vi "Main_MaintenanceCounters_V1.vi"() -> ()   [LabVIEW 2017]
panel:
  in  "LastCycleTimeCluster":cluster{"MachineName":string, "LastHour":string}
  out "LastCycleTimePath":path
  in  "CycleTimeArray":T1(array[cluster])
  in  "LastSeconds":i32
  out "ThisAppPath":path
  out "ModificationArray":string[](array[string])
  out "HourResetEnabled":string
  out "CycleCountHour":T2
  in  "ArrayCycleCountHour":T3(array[cluster])
  out "UserLevel":i32
  out "ServerConnectionStatus":string
  out "Line Name":string
  out "Array_BooleanMemoryPLC":T4(array[cluster])
  out "UserLogged":string
  in  "FormatCountersConfigArray":T5(array[cluster]) {"StoppageAlarmCounter" format="%#_6f"; "PreparationAlarmCounter" format="%#_6f"}
  out "CycleTimeCluster":T6
  out "Table Control":string[][](table)
  out "ConnectionCluster":cluster{"Connection":bool, "MachineName":string}
  out "UDT_1":T7
  in  "CountersConfiguration":T8
  out "CountersConfigMerged":T5(array[cluster])
  out "CounterLineName Path":path
  in  "Tab":T9(tab)
  in  "RefreshLists":bool
  in  "Selector_P#-Description":u16(ring) items=["104567 - Spinning Belt", "108724 - Emergency Stop", "105855 - Helicoil", "101415 - Inductive Sensor", "101111 - Magnetic Sensor"]
  in  "Selector_MachineSpareParts":u16(ring) items=["MA530", "MA520", "MA500-3", "MA500-2", "MA500-1", "MA490-2", "MA490-1", "MA475", "MA470", "MA455", "MA336", "MA335"]
  out "PathLocationMachineImage":path
  out "PathSparePartImage":path
  out "Image_LocationInMachine":T10(plugin-control)
  out "Image_SparePart":T10(plugin-control)
  in  "CountersConfigArray":T5(array[cluster]) {"StoppageAlarmCounter" format="%#_6f"; "PreparationAlarmCounter" format="%#_6f"}
  in  "RefreshCountersConfig":bool
  in  "SaveCountersConfig":bool
  out "Counters Configuration Path":path
  in  "MachineNameID":u16(ring) items=["MA530", "MA520", "MA500-3", "MA500-2", "MA500-1", "MA490-2", "MA490-1", "MA475", "MA470", "MA455", "MA336", "MA335"]
  in  "PLC Connection Array":T11(array[cluster]) {"PLC Type" items=["Keyence", "Allen Bradley", "Mitsubishi", "Panasonic", "Siemens"]}
  out "PLC Configuration Path":path
  in  "SavePLCConfig":bool
  in  "RefreshPLCConfig":bool
  in  "CreateTables":bool
  in  "EditUser":bool
  in  "GeneralParametersArray":cluster{"Parameter":string, "Value":string}[](array[cluster])
  in  "LoadDefaultConfig":bool
  in  "RemoveUser":bool
  in  "Logout":bool
  in  "Login":bool
  in  "AddUser":bool
  in  "GDrive":bool
  out "GeneralConfigPath":path
  in  "RefreshGeneralConfig":bool
  in  "SaveGeneralConfig":bool
  in  "ShowParetto":bool
  out "CycleTimeMonitor":T12(array[cluster])
  out "CycleTimePath":path
  out "legend":string[][](table)
  in  "Tab Control":T13(tab)
  in  "DictionaryArray":T14(array[cluster]) {"LifeCycle" format="%#_6f"}
  out "PathDictionary":path
  in  "SaveDictionary":bool
  in  "RefreshDictionary":bool
  in  "ResetAlarmButton":bool
  in  "QualityLogin":bool
  in  "MaintenanceLogin":bool
  in  "ResetAlarm":bool[](array[boolean])
  out "ArrayAlarm":bool[](array[boolean])
  out "OnlineStations":T15(array[cluster])
  in  "Counters Monitor Array":T16(array[cluster])
  out "CurrentCountersPath":path
  in  "Count Signal":bool[](array[boolean])
  in  "SaveCurrentCounter":bool
  in  "RefreshCurrentCounter":bool
  in  "Sort":bool
  out "Hour":string
  in  "stop":bool
  # "Cycles Based Maintenance"
  # "User"
  # "Line"
  # "Nidec Server Connection"
  # "Refresh Lists"
  # "Select Machine"
  # "Select PartNumber - Description"
  # "Location in the Machine"
  # "Spare Part Image"
  # "These paths are calculated automatically"
  # "Machine Name"
  # "Tool Crib P#"
  # "Description"
  # "SP1"
  # "SP2"
  # "Note:\nSP1 = Is the setpoint for the counter when the \nmachine will alert to prepare the replacement of\nthe component. This gives the technician time\nto get parts together.\n\nSP2 = Is the setpoint for the counter when the\nmachine will stop the operation until the part is \nreplaced, the operation can only be reset until\na quality employee comes to unlock with its \nuser and password."
  # "USER LEVEL 3 OR ABOVE TO ENABLE THIS CONFIGURATION IS NEEDED."
  # "Add the option to connect by serial port"
  # "Count Signal"
  # "Alarm Signal"
  # "Alarm Message"
  # "Machine Name"
  # "PLC Address"
  # "PLC Type"
  # "Value"
  # "Parameter"
  # "User Level 5 Requiered to View General Parameters"
  # "User Management"
  # "Idle Time: Is the maximum waiting time before a breakdown incidence is\nconsidered and created."
  # "Escalation Time: Is the maximum waiting time before sending an email \nto the escalation chain."
  # "Cycle Time Monitor"
  # "Cycle Time Monitor"
  # "Note: \nTo add a machine in this list of counters configuration it must be firt added in the PLC Connection tab."
  # "The SubAssembly can be either EOL, Motor, Stator, Rotor Etc, This is used to be able to crate several tables for the same line."
  # "buscar multiplos de ciclos para que coincidan \n\nestudiar investigacion de operaciones\n\nAgrupar las maquinas que trabajan en conjunto para agrupar tareas de mantenimiento.\nCambiar el metodo de seleccion de memorias de PLC usando solo strings para hacerlos universales."
  # "Nota para desarrollador: Revisar que al cerrar la incidencia se apague la alarma y se resetee el contador"
  # "1. Save counters to be loaded in the last state when the app starts up.\n\n2.Algorithm to read PLC counter values.\nthe key will be to set the signal from the PLC and reset from LabVIEW and the machine won't be able to start the new signal if the application has not been reset the previous one.\n\n3. Autosort getting the red status all the way up.\n\n4. Check cyle time between parts (The count signal must is the same for all the components in the same machine)"
  # "Component"
  # "Cycle Life"
  # "Manual"
  # "Un calculador de tiempo de vida en ciclos, que dependa del tipo de componente para calcular de acuerdo a la aplicacion.\n\npor ejemplo un slider, su tiempo de vida en es km de recorrido, midiendo cuanto se desplaza en cada movimiento, y cuantos desplazamientos hace por ciclo, se puede predecir, a los cuantos\nciclos va a fallar."
  # "Version:\nCBM V1.0\n03/03/2022 - 11:00\nEdgar Cruz\nMaintenance"
  # "MachineName"
  # "Tool Crib"
  # "ComponentName"
  # "Counter SetPoint"
  # "Actual"
  # "Status"
  # "Online Stations"
  # "Current Hour"
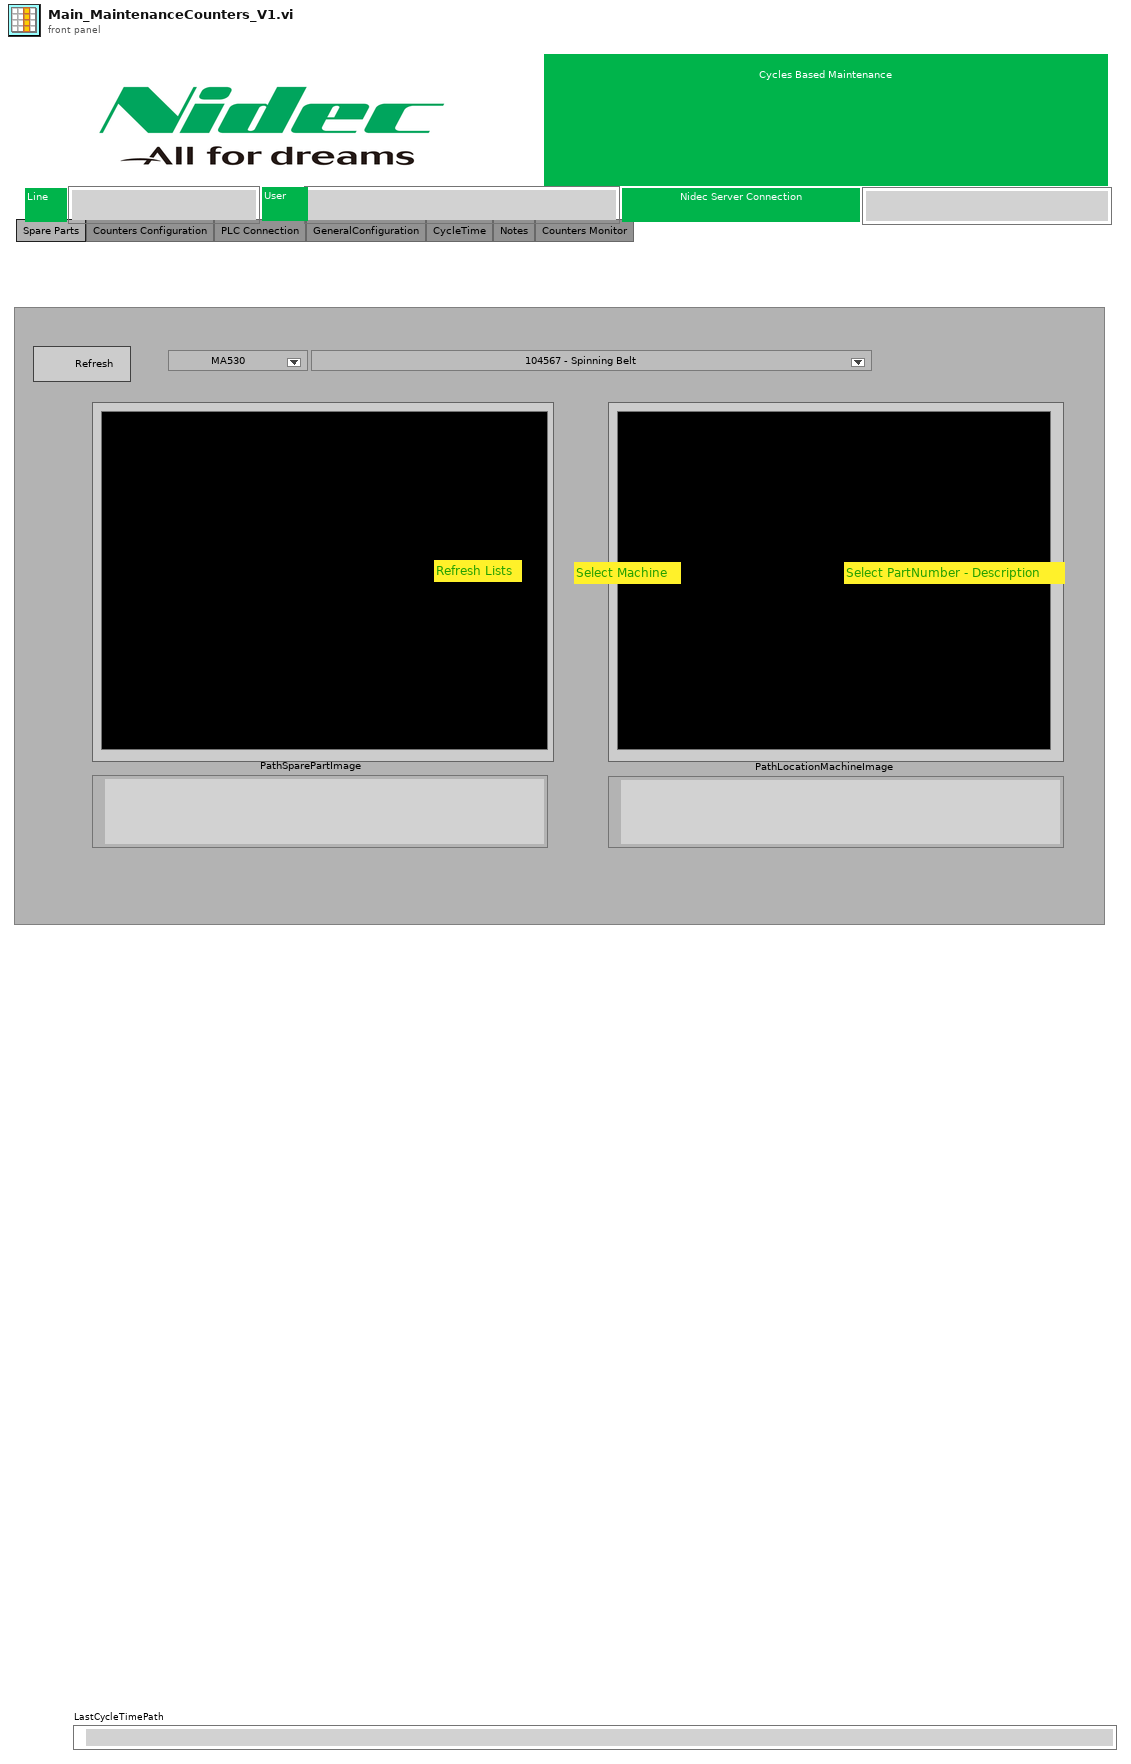
[diagram p1: front panel]
types:
  T1 = cluster{"MachineName":string, "LastHour":string}[]
  T2 = cluster{"MachineName":string, "HourLastCycle":string}
  T3 = cluster{"MachineName":string, "HourLastCycle":string}[]
  T4 = cluster{"PLC_Signal":bool, "MachineName":string}[]
  T5 = cluster{"ToolCribPartNumber":string, "ComponentName":string, "PreparationAlarmCounter":dbl, "StoppageAlarmCounter":dbl}[]
  T6 = cluster{"Connection":bool, "MachineName":string, "CycleTime":dbl}
  T7 = cluster{"ToolCribPartNumber":string, "ComponentName":string, "PreparationAlarmCounter":dbl, "StoppageAlarmCounter":dbl, "MachineName":string}
  T8 = cluster{"MachineName":string, "ComponentName":string, "StoppageAlarmCounter":dbl, "CurrentCount":dbl, "StatusColorBox":u32, "ToolCribPartNumber":string}
  T9 = enum32{"Spare Parts", "Counters Configuration", "PLC Connection", "GeneralConfiguration", "CycleTime", "Notes", "Counters Monitor"}
  T10 = typedef "IMAQ Image.ctl" = refnum<image>
  T11 = cluster{"MachineName":string, "PLC Address":string, "PLC Type":u16, "MemoryNumber1":string, "MemoryNumber2":string, "MemoryNumber3":string}[]
  T12 = cluster{"Connection":bool, "MachineName":string, "CycleTime":dbl}[]
  T13 = enum32{"Notes", "Dictionary", "Calculator", "Version Information"}
  T14 = cluster{"ComponentDescription":string, "LifeCycle":dbl, "ManualPDF":string}[]
  T15 = cluster{"Connection":bool, "MachineName":string}[]
  T16 = cluster{"MachineName":string, "ComponentName":string, "StoppageAlarmCounter":i32, "CurrentCount":i32, "StatusColorBox":u32, "ToolCribPartNumber":string}[]
  T17 = cluster{"ToolCribPartNumber":string, "ComponentName":string, "PreparationAlarmCounter":dbl, "StoppageAlarmCounter":dbl, "MachineName":string}[]
  T18 = cluster{"MachineName":string, "ComponentName":string, "StoppageAlarmCounter":i32, "CurrentCount":i32, "StatusColorBox":u32, "ToolCribPartNumber":string}
  T19 = enum8{"Enabled", "Disabled", "Disabled and Grayed Out"}
  T20 = typedef "Image Type" = u32
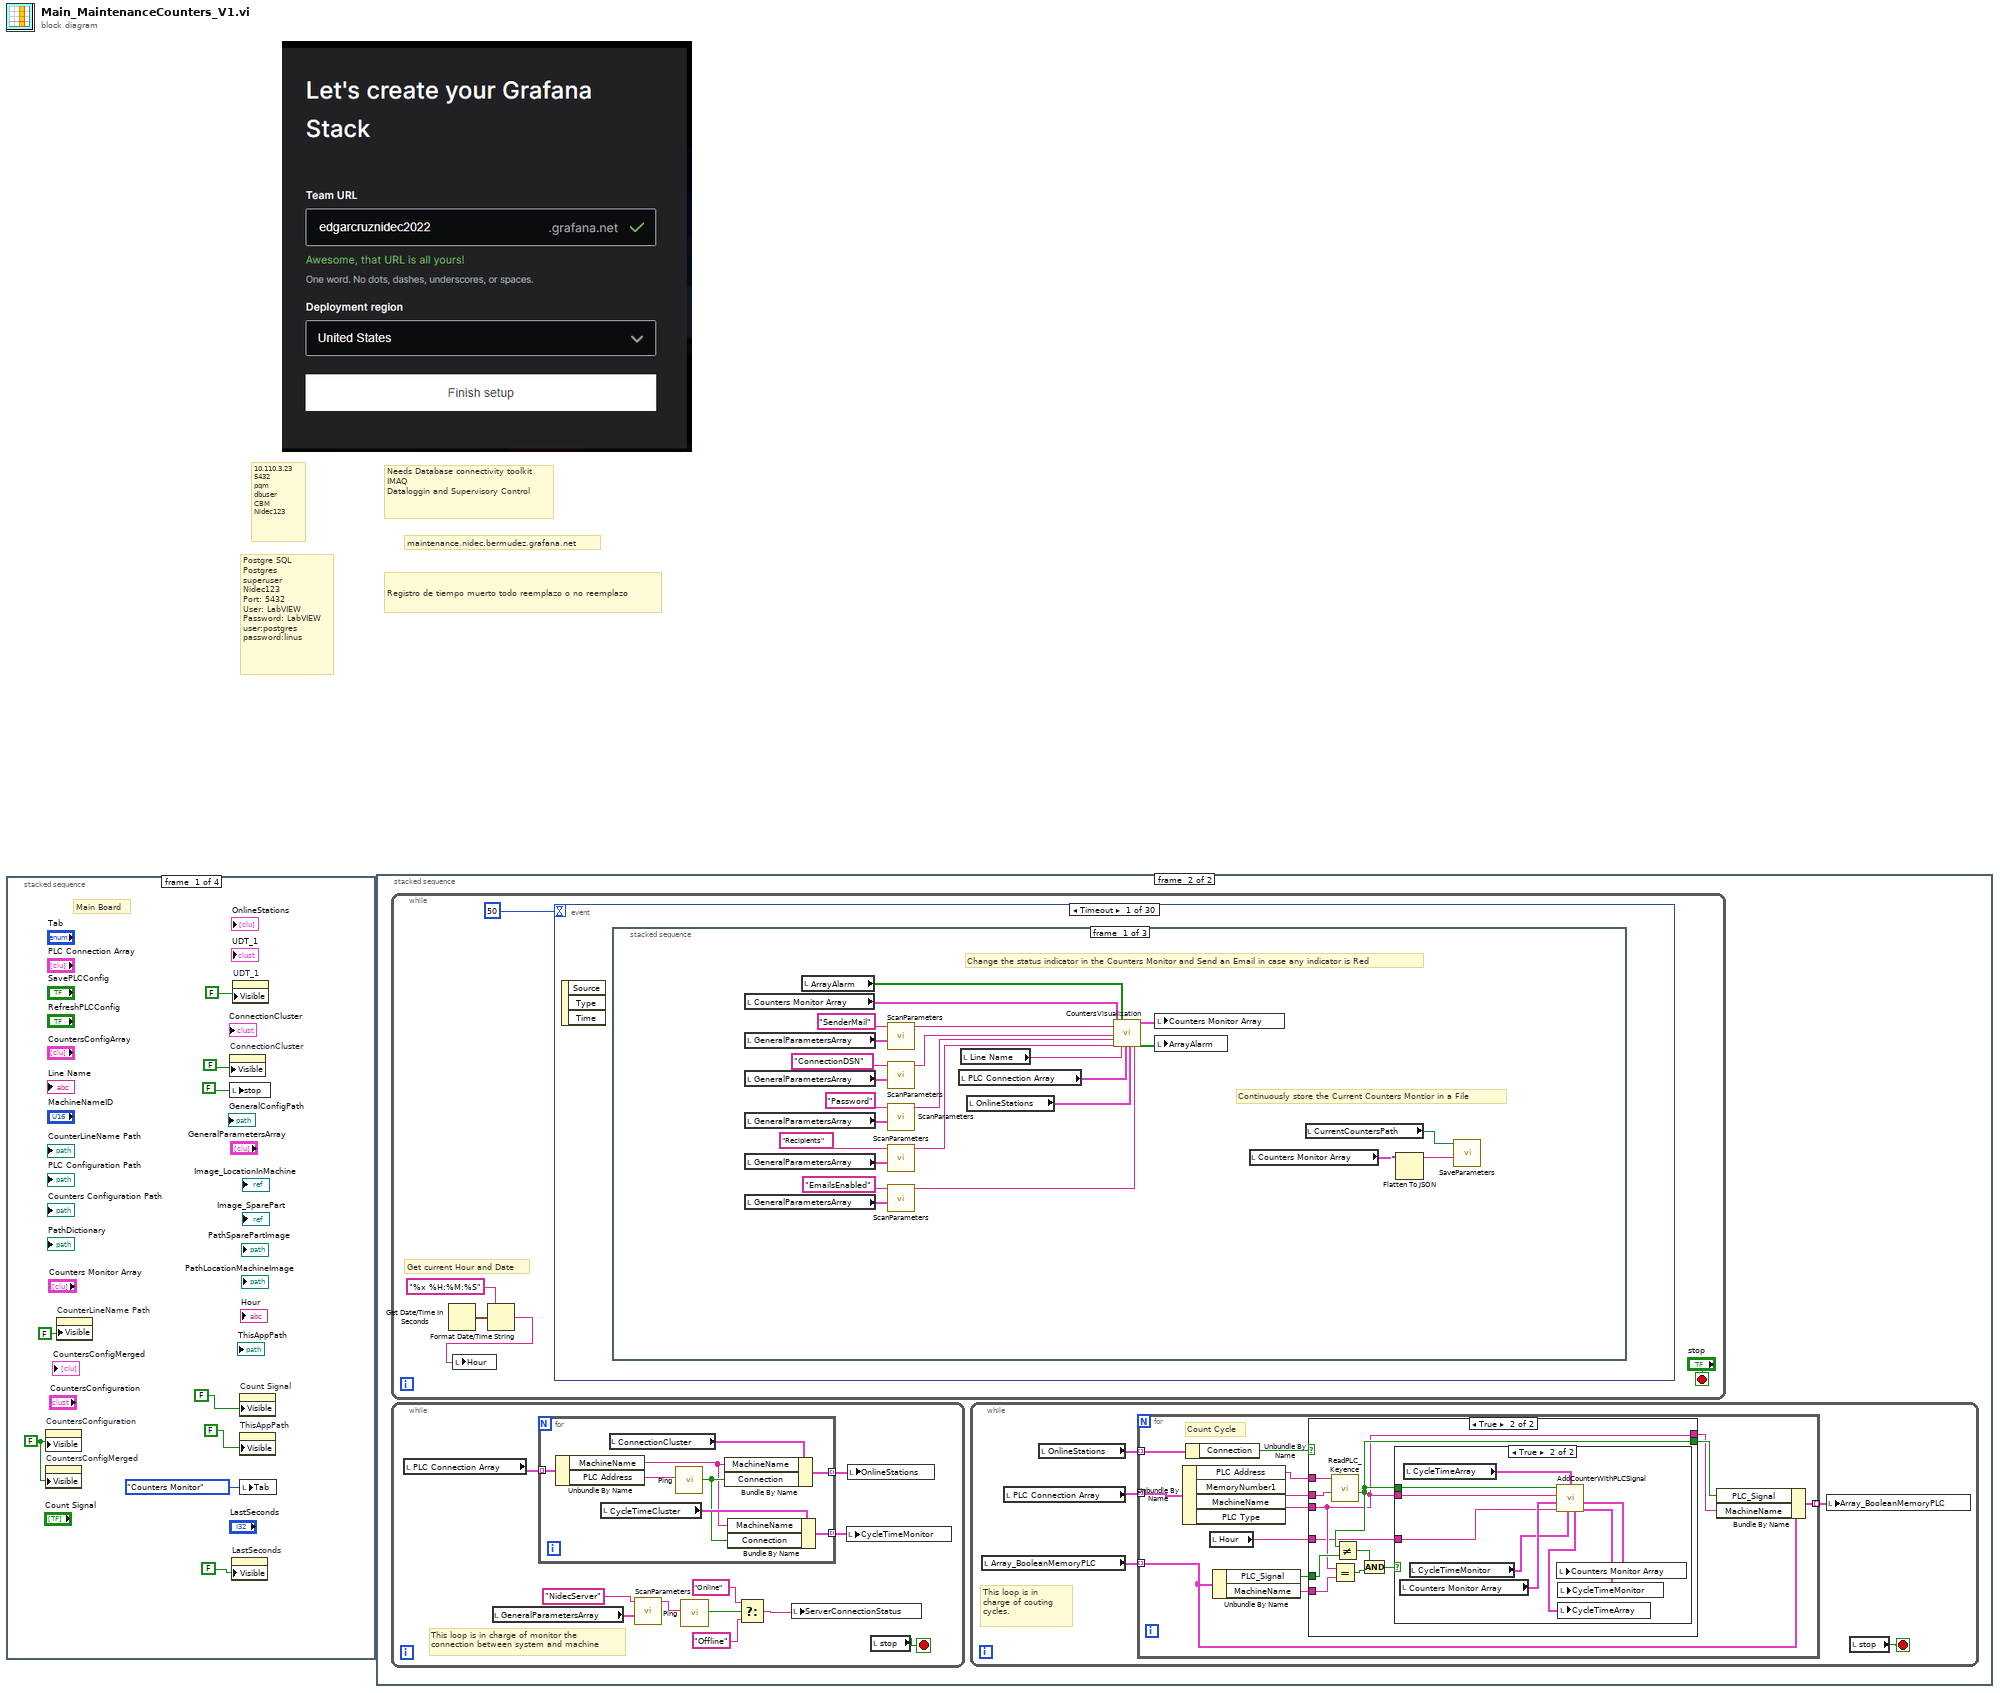
[diagram p0: block diagram]
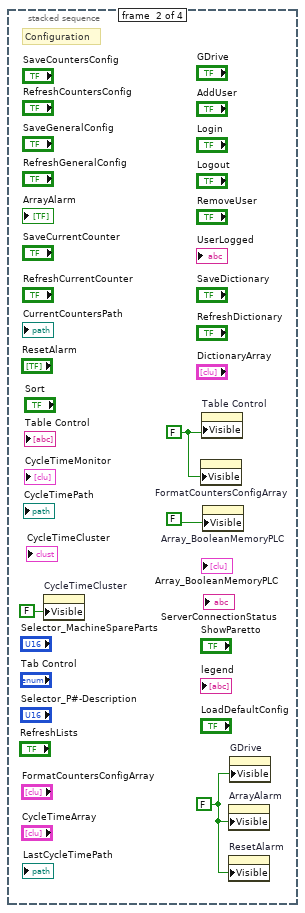
[diagram p2: hidden frame]
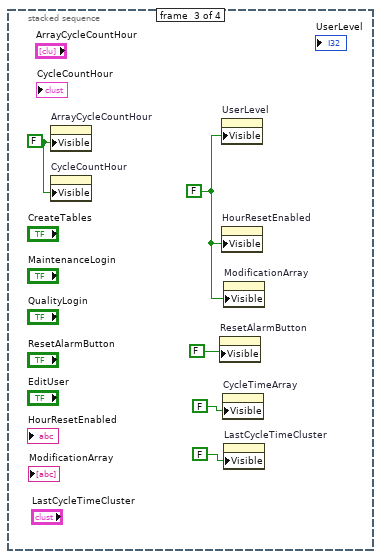
[diagram p3: hidden frame]
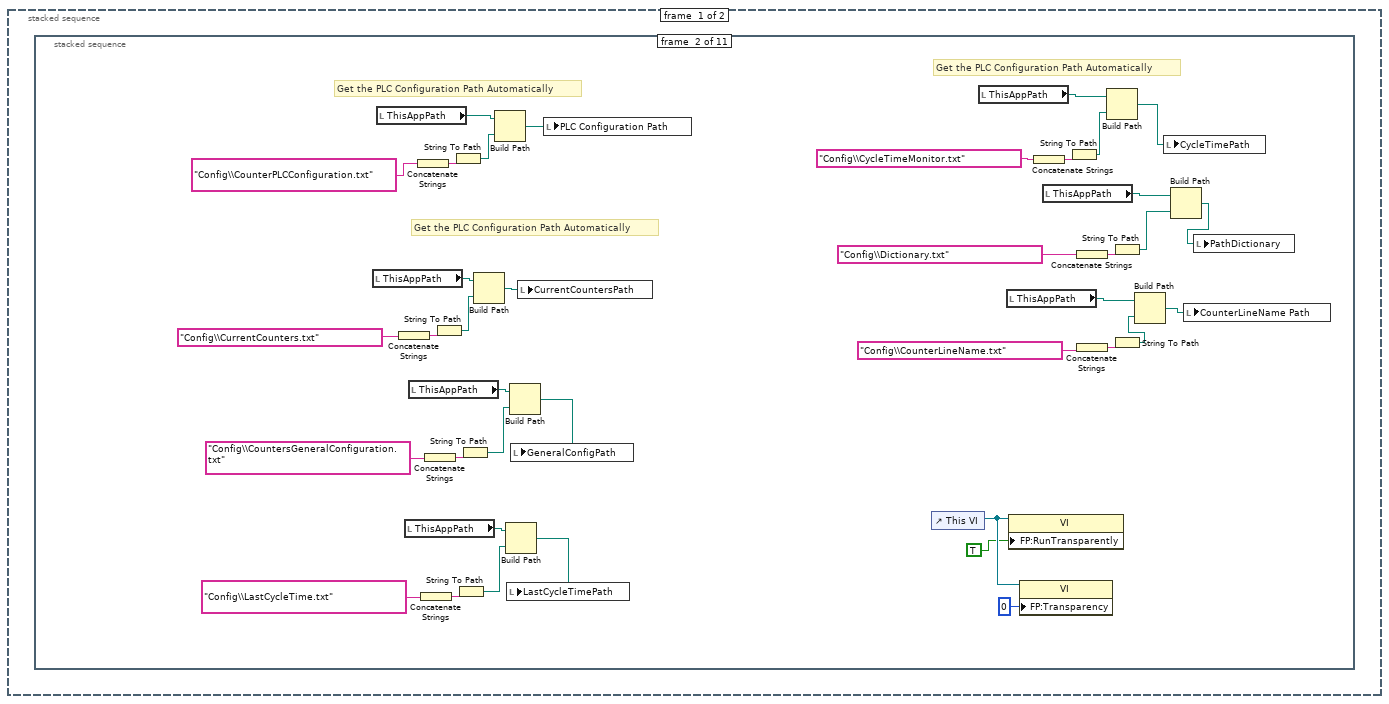
[diagram p5: hidden frame]
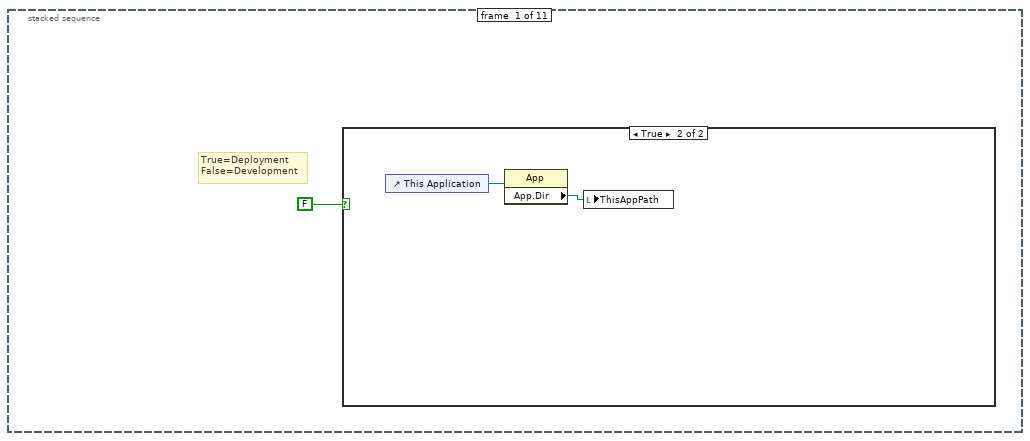
[diagram p6: hidden frame]
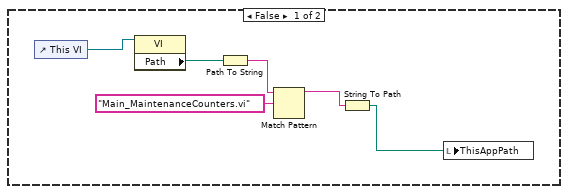
[diagram p7: hidden frame]
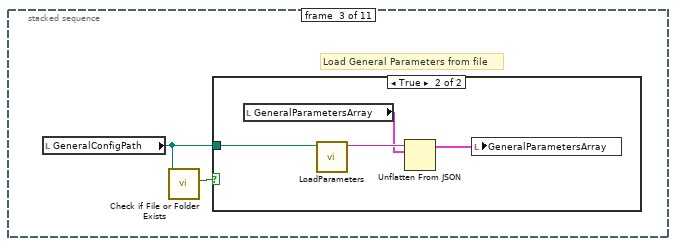
[diagram p8: hidden frame]
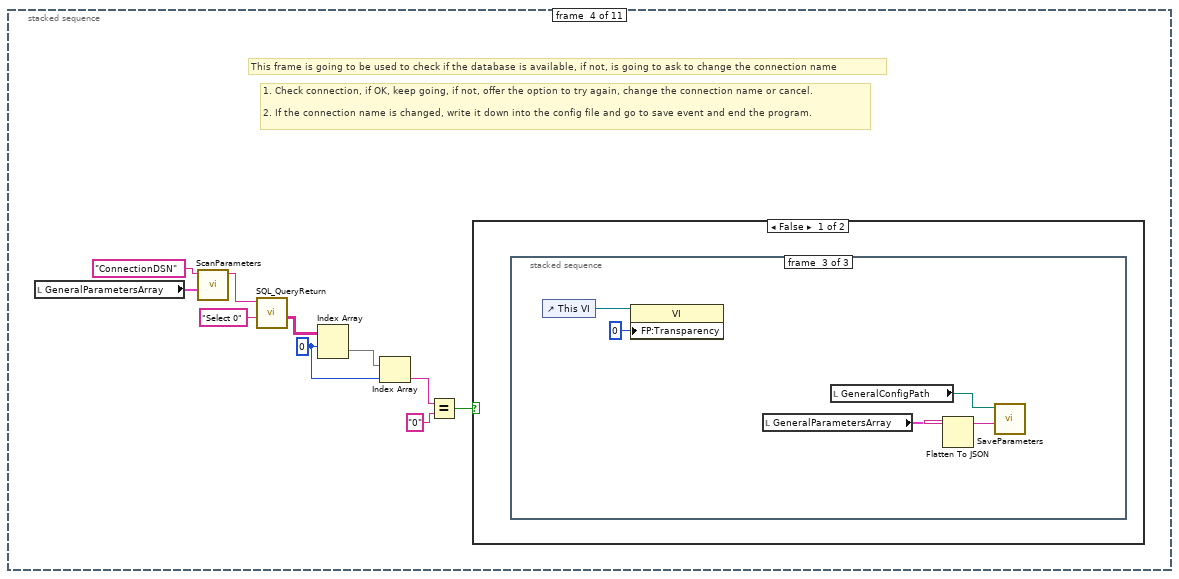
[diagram p10: hidden frame]
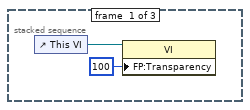
[diagram p11: hidden frame]
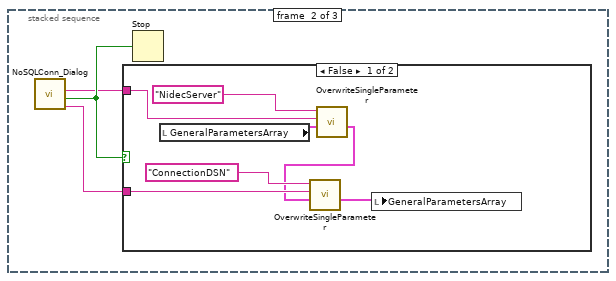
[diagram p12: hidden frame]
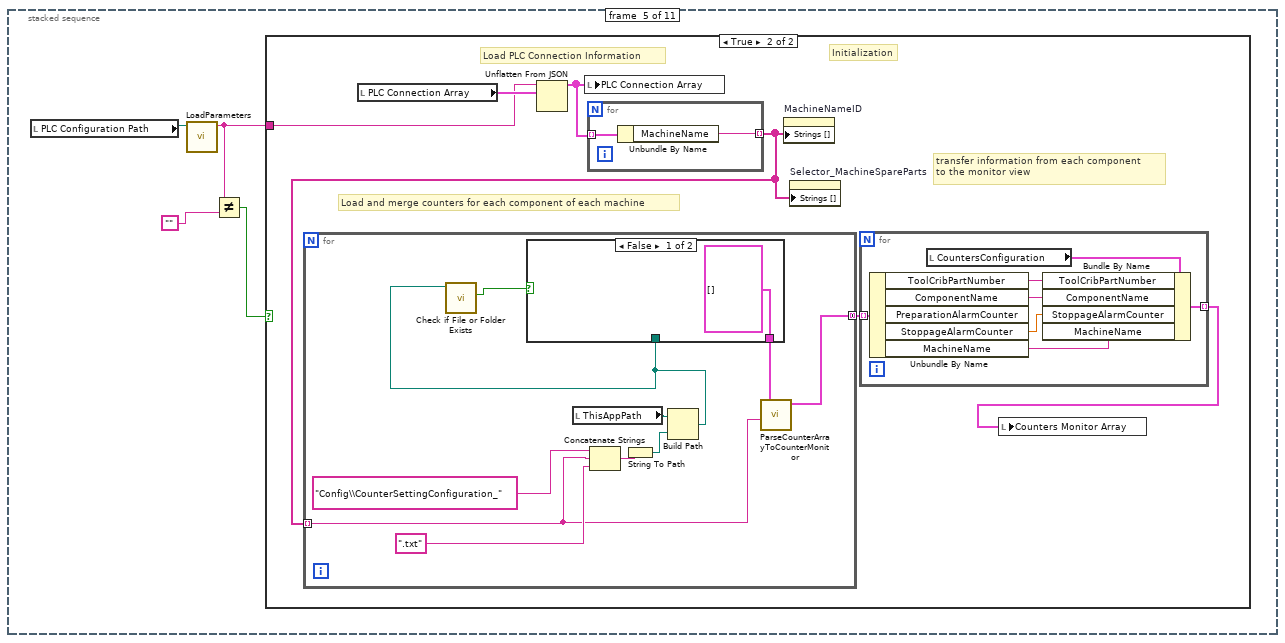
[diagram p15: hidden frame]
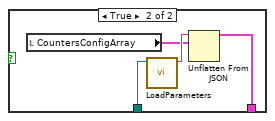
[diagram p17: hidden frame]
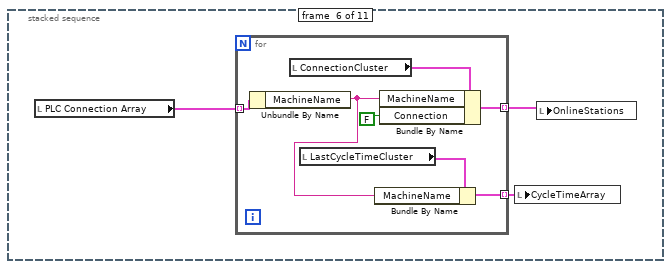
[diagram p18: hidden frame]
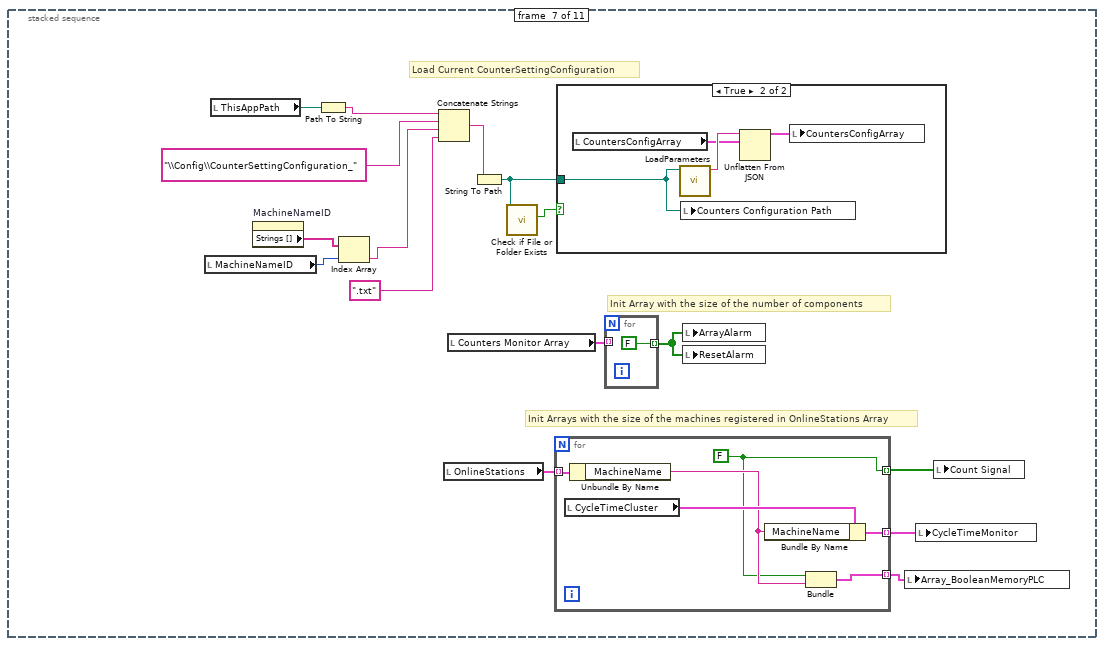
[diagram p19: hidden frame]
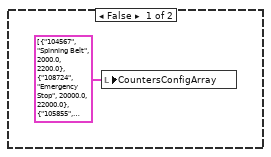
[diagram p20: hidden frame]
diagram:
  # "10.110.3.23\n5432\npqm\ndbuser\nCBM\nNidec123"
  # "maintenance.nidec.bermudez.grafana.net"
  # "Needs Database connectivity toolkit\nIMAQ\nDataloggin and Supervisory Control"
  # "Registro de tiempo muerto todo reemplazo o no reemplazo"
  # "Postgre SQL \nPostgres\nsuperuser\nNidec123\nPort: 5432\nUser: LabVIEW\nPassword: LabVIEW\nuser:postgres\npassword:linus"
  n1 = stacked-sequence {
    frame #0 {
      w8 = FALSE
      # "Main Board"
      n2 = property on="CountersConfiguration" class="Clust (strict)"("Visible"=w8) -> ()  [unwired: 2 in, 2 out]
      n3 = property on="CountersConfigMerged" class="Arr (strict)"("Visible"=w8) -> ()  [unwired: 2 in, 2 out]
      n4 = property on="CounterLineName Path" class="Path"("Visible"=FALSE) -> ()  [unwired: 2 in, 2 out]
      n5 = property on="ConnectionCluster" class="Clust (strict)"("Visible"=FALSE) -> ()  [unwired: 2 in, 2 out]
      n6 = local write "stop"(FALSE ("stop")) -> ()
      n7 = property on="LastSeconds" class="DigNum (strict)"("Visible"=FALSE) -> ()  [unwired: 2 in, 2 out]
      n8 = property on="UDT_1" class="Clust (strict)"("Visible"=FALSE) -> ()  [unwired: 2 in, 2 out]
      n9 = property on="Count Signal" class="Arr (strict)"("Visible"=FALSE) -> ()  [unwired: 2 in, 2 out]
      n10 = property on="ThisAppPath" class="Path"("Visible"=FALSE) -> ()  [unwired: 2 in, 2 out]
      n11 = local write "Tab"(T9."Counters Monitor" ("Tab")) -> ()
    }
    frame #1 {
      w11 = FALSE ("Visible")
      w12 = FALSE ("Visible")
      # "Configuration"
      n12 = property on="CycleTimeCluster" class="Clust (strict)"("Visible"=FALSE) -> ()  [unwired: 2 in, 2 out]
      n13 = property on="FormatCountersConfigArray" class="Arr (strict)"("Visible"=w12) -> ()  [unwired: 2 in, 2 out]
      n14 = property on="Table Control" class="Tbl (strict)"("Visible"=w12) -> ()  [unwired: 2 in, 2 out]
      n15 = property on="Array_BooleanMemoryPLC" class="Arr (strict)"("Visible"=FALSE) -> ()  [unwired: 2 in, 2 out]
      n16 = property on="ArrayAlarm" class="Arr (strict)"("Visible"=w11) -> ()  [unwired: 2 in, 2 out]
      n17 = property on="ResetAlarm" class="Arr (strict)"("Visible"=w11) -> ()  [unwired: 2 in, 2 out]
      n18 = property on="GDrive" class="Bool"("Visible"=w11) -> ()  [unwired: 2 in, 2 out]
    }
    frame #2 {
      w18 = FALSE
      w17 = FALSE
      n19 = property on="ArrayCycleCountHour" class="Arr (strict)"("Visible"=w18) -> ()  [unwired: 2 in, 2 out]
      n20 = property on="CycleCountHour" class="Clust (strict)"("Visible"=w18) -> ()  [unwired: 2 in, 2 out]
      n21 = property on="ResetAlarmButton" class="Bool"("Visible"=FALSE) -> ()  [unwired: 2 in, 2 out]
      n22 = property on="UserLevel" class="DigNum (strict)"("Visible"=w17) -> ()  [unwired: 2 in, 2 out]
      n23 = property on="HourResetEnabled" class="Str"("Visible"=w17) -> ()  [unwired: 2 in, 2 out]
      n24 = property on="CycleTimeArray" class="Arr (strict)"("Visible"=FALSE) -> ()  [unwired: 2 in, 2 out]
      n25 = property on="ModificationArray" class="Arr (strict)"("Visible"=w17) -> ()  [unwired: 2 in, 2 out]
      n26 = property on="LastCycleTimeCluster" class="Clust (strict)"("Visible"=FALSE) -> ()  [unwired: 2 in, 2 out]
    }
    frame #3 {
    }
  }
  n27 = stacked-sequence {
    frame #0 {
      n28 = stacked-sequence {
        frame #0 {
          # "True=Deployment\nFalse=Development"
          n29 = case shown="True" FALSE {
            frame False {
              n30 = control-ref of="This VI"() -> (w25:refnum<vi>)
              n31 = property class="VI"(reference=w25) -> ("Path"=w24:path)  [unwired: 1 in, 2 out]
              n32 = Path To String(path=w24) -> (string=w23:string)
              n33 = Match Pattern(string=w23, regular expression="Main_MaintenanceCounters.vi") -> (before substring=w21:string)  [unwired: 1 in, 3 out]
              n34 = String To Path(string=w21) -> (path=w20:path)
              n35 = local write "ThisAppPath"(w20) -> ()
            }
            frame True {
              n36 = control-ref of="This Application"() -> (w27:refnum<vi>)
              n37 = property class="App"(reference=w27) -> ("App.Dir"=w26:path)  [unwired: 1 in, 2 out]
              n38 = local write "ThisAppPath"(w26) -> ()
            }
          }
        }
        frame #1 {
          # "Get the PLC Configuration Path Automatically"
          # "Get the PLC Configuration Path Automatically"
          # "Get the PLC Configuration Path Automatically"
          n39 = local read "ThisAppPath"() -> (w47:path)
          n40 = local read "ThisAppPath"() -> (w49:path)
          n41 = Concatenate Strings("Config\\CurrentCounters.txt" ("regular expression")) -> (w62:string)
          n42 = local read "ThisAppPath"() -> (w30:path)
          n43 = local read "ThisAppPath"() -> (w44:path)
          n44 = Concatenate Strings("Config\\CounterPLCConfiguration.txt" ("regular expression")) -> (w65:string)
          n45 = Concatenate Strings("Config\\LastCycleTime.txt" ("regular expression")) -> (w28:string)
          n46 = Concatenate Strings("Config\\CountersGeneralConfiguration.txt" ("regular expression")) -> (w57:string)
          n47 = String To Path(string=w62) -> (path=w46:path)
          n48 = String To Path(string=w65) -> (path=w50:path)
          n49 = String To Path(string=w28) -> (path=w31:path)
          n50 = String To Path(string=w57) -> (path=w43:path)
          n51 = Build Path(base path=w47, name or relative path=w46) -> (appended path=w45:path)
          n52 = Build Path(base path=w49, name or relative path=w50) -> (appended path=w48:path)
          n53 = Build Path(base path=w30, name or relative path=w31) -> (appended path=w32:path)
          n54 = local write "LastCycleTimePath"(w32) -> ()
          n55 = Build Path(base path=w44, name or relative path=w43) -> (appended path=w42:path)
          n56 = local write "GeneralConfigPath"(w42) -> ()
          n57 = local write "CurrentCountersPath"(w45) -> ()
          n58 = local write "PLC Configuration Path"(w48) -> ()
          n59 = control-ref of="This VI"() -> (w53:refnum<vi>)
          n60 = local read "ThisAppPath"() -> (w41:path)
          n61 = local read "ThisAppPath"() -> (w35:path)
          n62 = property class="VI"(reference=w53, "FP:RunTransparently"=TRUE) -> ()  [unwired: 1 in, 2 out]
          n63 = property class="VI"(reference=w53, "FP:Transparency"=u8 0 ("Front Panel Window:Transparency")) -> ()  [unwired: 1 in, 2 out]
          n64 = Concatenate Strings("Config\\CycleTimeMonitor.txt" ("regular expression")) -> (w61:string)
          n65 = local read "ThisAppPath"() -> (w38:path)
          n66 = String To Path(string=w61) -> (path=w40:path)
          n67 = Concatenate Strings("Config\\Dictionary.txt" ("regular expression")) -> (w58:string)
          n68 = Concatenate Strings("Config\\CounterLineName.txt" ("regular expression")) -> (w55:string)
          n69 = Build Path(base path=w41, name or relative path=w40) -> (appended path=w39:path)
          n70 = String To Path(string=w58) -> (path=w37:path)
          n71 = String To Path(string=w55) -> (path=w34:path)
          n72 = Build Path(base path=w35, name or relative path=w34) -> (appended path=w33:path)
          n73 = local write "CycleTimePath"(w39) -> ()
          n74 = Build Path(base path=w38, name or relative path=w37) -> (appended path=w36:path)
          n75 = local write "CounterLineName Path"(w33) -> ()
          n76 = local write "PathDictionary"(w36) -> ()
        }
        frame #2 {
          # "Load General Parameters from file"
          n77 = local read "GeneralConfigPath"() -> (w66:path)
          n78 = call <vilib>:"Check if File or Folder Exists.vi"("path"=w66) -> ("file or folder exists?"=w67:bool)  [unwired: 8 in, 2 out]
          n79 = case shown="True" w67 {
            tunnel: w66 -> [_ w71]
            frame False {
            }
            frame True {
              n80 = local read "GeneralParametersArray"() -> (w69:cluster{"Parameter":string, "Value":string}[])
              n81 = call "LoadParameters.vi"("ShiftConfigPath"=w71) -> ("JSON_Text"=w70:string)  [unwired: 10 in]
              n82 = Unflatten From JSON(JSON string=w70, type and defaults=w69) -> (value=w68:cluster{"Parameter":string, "Value":string}[])  [unwired: 5 in, 1 out]
              n83 = local write "GeneralParametersArray"(w68) -> ()
            }
          }
        }
        frame #3 {
          w74 = 0 ("index (row)")
          # "1. Check connection, if OK, keep going, if not, offer the option to try again, change the connection name or cancel.\n\n2. If the connection name is changed, write it down into the config file and go to save event and end the program."
          # "This frame is going to be used to check if the database is available, if not, is going to ask to change the connection name"
          n84 = local read "GeneralParametersArray"() -> (w81:cluster{"Parameter":string, "Value":string}[])
          n85 = call "ScanParameters.vi"("MainConfigurationArray"=w81, "Parameter"="ConnectionDSN") -> ("Value"=w79:string)  [unwired: 9 in]
          n86 = call "SQL_QueryReturn.vi"("SQL query"="Select 0", "ConnectionDSN"=w79) -> ("data"=w77:string[][])  [unwired: 9 in]
          n87 = Index Array(array=w77, index (row)=w74) -> (element=w75:string[])  [unwired: 1 in]
          n88 = Index Array(array=w75, index=w74) -> (element=w73:string)
          n89 = Equal?(x=w73, y="0" ("SQL query")) -> (x = y?=w72:bool)
          n90 = case shown="False" w72 {
            frame False {
              n91 = stacked-sequence {
                frame #0 {
                  n92 = control-ref of="This VI"() -> (w82:refnum<vi>)
                  n93 = property class="VI"(reference=w82, "FP:Transparency"=u8 100 ("Front Panel Window:Transparency")) -> ()  [unwired: 1 in, 2 out]
                }
                frame #1 {
                  n94 = call "NoSQLConn_Dialog.vi"() -> ("NewDSN"=w86:string, "Boolean"=w85:bool, "NewIPAddress"=w84:string)  [unwired: 9 in]
                  n95 = case shown="False" w85 {
                    tunnel: w86 -> [w92 _]
                    tunnel: w84 -> [w89 _]
                    frame False {
                      n96 = local read "GeneralParametersArray"() -> (w90:cluster{"Parameter":string, "Value":string}[])
                      n97 = call "OverwriteSingleParameter.vi"("MainConfigurationArrayIN"=w90, "Value"=w89, "Parameter"="NidecServer") -> ("MainConfigurationArrayOUT"=w87:cluster{"Parameter":string, "Value":string}[])  [unwired: 8 in]
                      n98 = call "OverwriteSingleParameter.vi"("MainConfigurationArrayIN"=w87, "Value"=w92, "Parameter"="ConnectionDSN") -> ("MainConfigurationArrayOUT"=w88:cluster{"Parameter":string, "Value":string}[])  [unwired: 8 in]
                      n99 = local write "GeneralParametersArray"(w88) -> ()
                    }
                    frame True {
                    }
                  }
                  n100 = Stop(stop? (T)=w85) -> ()
                }
                frame #2 {
                  n101 = control-ref of="This VI"() -> (w98:refnum<vi>)
                  n102 = property class="VI"(reference=w98, "FP:Transparency"=u8 0 ("Front Panel Window:Transparency")) -> ()  [unwired: 1 in, 2 out]
                  n103 = local read "GeneralParametersArray"() -> (w94:cluster{"Parameter":string, "Value":string}[])
                  n104 = local read "GeneralConfigPath"() -> (w96:path)
                  n105 = Flatten To JSON(anything=w94) -> (JSON string=w95:string)  [unwired: 2 in, 1 out]
                  n106 = call "SaveParameters.vi"("JSON_Text"=w95, "ShiftConfigPath"=w96) -> ()  [unwired: 10 in]
                }
              }
            }
            frame True {
            }
          }
        }
        frame #4 {
          n107 = local read "PLC Configuration Path"() -> (w102:path)
          n108 = call "LoadParameters.vi"("ShiftConfigPath"=w102) -> ("JSON_Text"=w101:string)  [unwired: 10 in]
          n109 = Not Equal?(x=w101, y="") -> (x != y?=w99:bool)
          n110 = case shown="True" w99 {
            tunnel: w101 -> [_ w103]
            frame False {
            }
            frame True {
              # "Initialization"
              # "transfer information from each component\nto the monitor view"
              # "Load and merge counters for each component of each machine"
              # "Load PLC Connection Information"
              n111 = local read "PLC Connection Array"() -> (w108:T11)
              n112 = Unflatten From JSON(JSON string=w103, type and defaults=w108) -> (value=w107:T11)  [unwired: 5 in, 1 out]
              n113 = local write "PLC Connection Array"(w107) -> ()
              n114 = for {
                tunnel: w107 -> [w131] mode=indexing
                tunnel: [w132] -> w104 mode=indexing
                n115 = Unbundle By Name(w131) -> ("MachineName"=w132:string)
              }
              n116 = for {
                tunnel: w104 -> [w122] mode=indexing
                tunnel: [w121] -> w105 mode=concatenating
                n117 = local read "ThisAppPath"() -> (w118:path)
                n118 = Concatenate Strings("Config\\CounterSettingConfiguration_" ("regular expression"), w122, ".txt" ("regular expression")) -> (w125:string)
                n119 = String To Path(string=w125) -> (path=w117:path)
                n120 = Build Path(base path=w118, name or relative path=w117) -> (appended path=w116:path)
                n121 = call <vilib>:"Check if File or Folder Exists.vi"("path"=w116) -> ("file or folder exists?"=w120:bool)  [unwired: 8 in, 2 out]
                n122 = case shown="False" w120 {
                  tunnel: [T5 [] ("CountersConfigArray") w129] -> w119
                  tunnel: w116 -> [_ w128]
                  frame False {
                  }
                  frame True {
                    n123 = local read "CountersConfigArray"() -> (w127:T5)
                    n124 = call "LoadParameters.vi"("ShiftConfigPath"=w128) -> ("JSON_Text"=w130:string)  [unwired: 10 in]
                    n125 = Unflatten From JSON(JSON string=w130, type and defaults=w127) -> (value=w129:T5)  [unwired: 5 in, 1 out]
                  }
                }
                n126 = call "ParseCounterArrayToCounterMonitor.vi"("MachineID"=w122, "CountersConfigArray"=w119) -> ("CounterMonitorArray"=w121:T17)  [unwired: 9 in]
              }
              n127 = property on="MachineNameID" class="Ring (strict)"("Strings []"=w104) -> ()  [unwired: 2 in, 2 out]
              n128 = property on="Selector_MachineSpareParts" class="Ring (strict)"("Strings []"=w104) -> ()  [unwired: 2 in, 2 out]
              n129 = for {
                tunnel: [w113] -> w106 mode=indexing
                tunnel: w105 -> [w112] mode=indexing
                n130 = Unbundle By Name(w112) -> ("ToolCribPartNumber"=w111:string, "ComponentName"=w114:string, "StoppageAlarmCounter"=w110:dbl, "MachineName"=w109:string)  [unwired: 1 out]
                n131 = local read "CountersConfiguration"() -> (w115:T8)
                n132 = Bundle By Name(cluster=w115, "ToolCribPartNumber"=w111, "ComponentName"=w114, "StoppageAlarmCounter"=w110, "MachineName"=w109) -> (w113:T8)
              }
              n133 = local write "Counters Monitor Array"(w106) -> ()
            }
          }
        }
        frame #5 {
          n134 = local read "PLC Connection Array"() -> (w135:T11)
          n135 = for {
            tunnel: w135 -> [w142] mode=indexing
            tunnel: [w140] -> w134 mode=indexing
            tunnel: [w136] -> w133 mode=indexing
            n136 = Unbundle By Name(w142) -> ("MachineName"=w137:string)
            n137 = local read "ConnectionCluster"() -> (w141:cluster{"Connection":bool, "MachineName":string})
            n138 = local read "LastCycleTimeCluster"() -> (w138:cluster{"MachineName":string, "LastHour":string})
            n139 = Bundle By Name(cluster=w138, "MachineName"=w137) -> (w136:cluster{"MachineName":string, "LastHour":string})
            n140 = Bundle By Name(cluster=w141, "MachineName"=w137, "Connection"=FALSE) -> (w140:cluster{"Connection":bool, "MachineName":string})
          }
          n141 = local write "CycleTimeArray"(w133) -> ()
          n142 = local write "OnlineStations"(w134) -> ()
        }
        frame #6 {
          # "Load Current CounterSettingConfiguration"
          # "Init Array with the size of the number of components"
          # "Init Arrays with the size of the machines registered in OnlineStations Array"
          n143 = local read "MachineNameID"() -> (w158:u16)
          n144 = local read "ThisAppPath"() -> (w143:path)
          n145 = property on="MachineNameID" class="Ring (strict)"() -> ("Strings []"=w157:string[])  [unwired: 2 in, 2 out]
          n146 = Path To String(path=w143) -> (string=w144:string)
          n147 = Index Array(array=w157, index=w158) -> (element=w155:string)
          n148 = Concatenate Strings(w144, "\\Config\\CounterSettingConfiguration_" ("regular expression"), w155, ".txt" ("regular expression")) -> (w156:string)
          n149 = local read "OnlineStations"() -> (w148:T15)
          n150 = local read "Counters Monitor Array"() -> (w150:T16)
          n151 = String To Path(string=w156) -> (path=w153:path)
          n152 = call <vilib>:"Check if File or Folder Exists.vi"("path"=w153) -> ("file or folder exists?"=w154:bool)  [unwired: 8 in, 2 out]
          n153 = for {
            tunnel: w148 -> [w163] mode=indexing
            tunnel: [w160] -> w147 mode=indexing
            tunnel: [w162] -> w146 mode=indexing
            tunnel: [w159] -> w145 mode=indexing
            w160 = FALSE
            n154 = local read "CycleTimeCluster"() -> (w164:T6)
            n155 = Unbundle By Name(w163) -> ("MachineName"=w161:string)
            n156 = Bundle By Name(cluster=w164, "MachineName"=w161) -> (w162:T6)
            n157 = Bundle(w160, "MachineName"=w161) -> (w159:cluster{bool, "MachineName":string})  [unwired: 1 in]
          }
          n158 = case shown="True" w154 {
            tunnel: w153 -> [_ w169]
            frame False {
              n159 = local write "CountersConfigArray"(T5 [{"ToolCribPartNumber"="104567", "ComponentName"="Spinning Belt", "PreparationAlarmCounter"=2000.0, "StoppageAlarmCounter"=2200.0}, {"ToolCribPartNumber"="108724", "ComponentName"="Emergency Stop", "PreparationAlarmCounter"=20000.0, "StoppageAlarmCounter"=22000.0}, {"ToolCribPartNumber"="105855", "ComponentName"="Helicoil", "PreparationAlarmCounter"=38000.0, "StoppageAlarmCounter"=40000.0}, {"ToolCribPartNumber"="101415", "ComponentName"="NewPart", "PreparationAlarmCounter"=12000.0, "StoppageAlarmCounter"=12300.0}] ("CountersConfigArray")) -> ()
            }
            frame True {
              n160 = local read "CountersConfigArray"() -> (w168:T5)
              n161 = call "LoadParameters.vi"("ShiftConfigPath"=w169) -> ("JSON_Text"=w170:string)  [unwired: 10 in]
              n162 = local write "Counters Configuration Path"(w169) -> ()
              n163 = Unflatten From JSON(JSON string=w170, type and defaults=w168) -> (value=w167:T5)  [unwired: 5 in, 1 out]
              n164 = local write "CountersConfigArray"(w167) -> ()
            }
          }
          n165 = for {
            tunnel: w150 -> [_] mode=indexing
            tunnel: [FALSE] -> w149 mode=indexing
          }
          n166 = local write "ArrayAlarm"(w149) -> ()
          n167 = local write "ResetAlarm"(w149) -> ()
          n168 = local write "Array_BooleanMemoryPLC"(w145) -> ()
          n169 = local write "CycleTimeMonitor"(w146) -> ()
          n170 = local write "Count Signal"(w147) -> ()
        }
        frame #7 {
          # "Load Dictionary"
          n171 = local read "CurrentCountersPath"() -> (w177:path)
          n172 = local read "Counters Monitor Array"() -> (w175:T16)
          n173 = local read "PathDictionary"() -> (w171:path)
          n174 = call "LoadParameters.vi"("ShiftConfigPath"=w177) -> ("JSON_Text"=w176:string)  [unwired: 10 in]
          n175 = call <vilib>:"Check if File or Folder Exists.vi"("path"=w171) -> ("file or folder exists?"=w172:bool)  [unwired: 8 in, 2 out]
          n176 = Unflatten From JSON(JSON string=w176, type and defaults=w175) -> (value=w174:T16)  [unwired: 5 in, 1 out]
          n177 = for {
            tunnel: w175 -> [w183] mode=indexing
            tunnel: w174 -> [w184]
            tunnel: [w182] -> w173 mode=indexing
            n178 = Unbundle By Name(w183) -> ("MachineName"=w187:string, "ComponentName"=w186:string, "ToolCribPartNumber"=w185:string)
            n179 = for {
              tunnel: w187 -> [w200]
              tunnel: w186 -> [w199]
              tunnel: w185 -> [w198]
              tunnel: w184 -> [w201] mode=indexing
              shift-right: [w188] -> w182
              shift-left: w183 -> [w189]
              n180 = Unbundle By Name(w201) -> ("MachineName"=w190:string, "ComponentName"=w191:string, "ToolCribPartNumber"=w192:string, "CurrentCount"=w194:i32)
              n181 = Equal?(x=w200, y=w190) -> (x = y?=w196:bool)
              n182 = Equal?(x=w199, y=w191) -> (x = y?=w197:bool)
              n183 = Equal?(x=w198, y=w192) -> (x = y?=w195:bool)
              n184 = Compound Arithmetic op=AND(w196, w197, w195) -> (w193:bool)
              n185 = case shown="True" w193 {
                tunnel: w194 -> [_ w208]
                tunnel: w192 -> [_ w207]
                tunnel: w191 -> [_ w206]
                tunnel: w190 -> [_ w205]
                tunnel: w189 -> [w202 w204]
                tunnel: [w202 w203] -> w188
                frame False {
                }
                frame True {
                  n186 = Bundle By Name(cluster=w204, "MachineName"=w205, "ComponentName"=w206, "ToolCribPartNumber"=w207, "CurrentCount"=w208) -> (w203:T18)
                }
              }
            }
          }
          n187 = case shown="True" w172 {
            tunnel: w171 -> [_ w180]
            frame False {
            }
            frame True {
              n188 = local read "DictionaryArray"() -> (w181:T14)
              n189 = call "LoadParameters.vi"("ShiftConfigPath"=w180) -> ("JSON_Text"=w179:string)  [unwired: 10 in]
              n190 = Unflatten From JSON(JSON string=w179, type and defaults=w181) -> (value=w178:T14)  [unwired: 5 in, 1 out]
              n191 = local write "DictionaryArray"(w178) -> ()
            }
          }
          n192 = local write "Counters Monitor Array"(w173) -> ()
        }
        frame #8 {
          w213 = T19."Disabled and Grayed Out" ("Disabled")
          # "Logout and disable information"
          # "Load Line name from General parameters"
          n193 = local write "UserLevel"(0) -> ()
          n194 = local write "UserLogged"("") -> ()
          n195 = property on="PLC Connection Array" class="Arr (strict)"("DisabledEnum"=w213) -> ()  [unwired: 2 in, 2 out]
          n196 = property on="GeneralParametersArray" class="Arr (strict)"("Visible"=FALSE) -> ()  [unwired: 2 in, 2 out]
          n197 = property on="CountersConfigArray" class="Arr (strict)"("DisabledEnum"=w213) -> ()  [unwired: 2 in, 2 out]
          n198 = local read "GeneralParametersArray"() -> (w210:cluster{"Parameter":string, "Value":string}[])
          n199 = call "ScanParameters.vi"("MainConfigurationArray"=w210, "Parameter"="LineName") -> ("Value"=w211:string)  [unwired: 9 in]
          n200 = local write "Line Name"(w211) -> ()
        }
        frame #9 {
          # "This array must have one element per machine and register the hour \nso it must be initialized with the number of stations"
          n201 = local read "OnlineStations"() -> (w231:T15)
          n202 = for {
            tunnel: w231 -> [w235] mode=indexing
            tunnel: [w232] -> w230 mode=indexing
            n203 = Unbundle By Name(w235) -> ("MachineName"=w233:string)
            n204 = local read "CycleCountHour"() -> (w234:T2)
            n205 = Bundle By Name(cluster=w234, "MachineName"=w233) -> (w232:T2)
          }
          n206 = local read "GeneralParametersArray"() -> (w223:cluster{"Parameter":string, "Value":string}[])
          n207 = local read "GeneralParametersArray"() -> (w222:cluster{"Parameter":string, "Value":string}[])
          n208 = local write "ArrayCycleCountHour"(w230) -> ()
          n209 = local read "GeneralParametersArray"() -> (w228:cluster{"Parameter":string, "Value":string}[])
          n210 = call "ScanParameters.vi"("MainConfigurationArray"=w223, "Parameter"="LineName") -> ("Value"=w224:string)  [unwired: 9 in]
          n211 = call "ScanParameters.vi"("MainConfigurationArray"=w222, "Parameter"="SubAssembly") -> ("Value"=w225:string)  [unwired: 9 in]
          n212 = Concatenate Strings("update \"", w224, "_userlogged\" set \"useroperations\"='0',\"userquality\"='0' where \"subassembly\"='", w225, "'") -> (w226:string)
          n213 = call "ScanParameters.vi"("MainConfigurationArray"=w228, "Parameter"="ConnectionDSN") -> ("Value"=w229:string)  [unwired: 9 in]
          n214 = To Lower Case(string=w226) -> (all lower case string=w227:string)
          n215 = call "SQL_QueryNoReturn.vi"("SQL query"=w227, "ConnectionDSN"=w229) -> ()  [unwired: 10 in]
        }
        frame #10 {
          n216 = local read "GeneralParametersArray"() -> (w239:cluster{"Parameter":string, "Value":string}[])
          n217 = local read "GeneralParametersArray"() -> (w241:cluster{"Parameter":string, "Value":string}[])
          n218 = local read "GeneralParametersArray"() -> (w245:cluster{"Parameter":string, "Value":string}[])
          n219 = local read "Counters Monitor Array"() -> (w236:T16)
          n220 = call "ScanParameters.vi"("MainConfigurationArray"=w239, "Parameter"="SubAssembly") -> ("Value"=w237:string)  [unwired: 9 in]
          n221 = call "ScanParameters.vi"("MainConfigurationArray"=w241, "Parameter"="LineName") -> ("Value"=w240:string)  [unwired: 9 in]
          n222 = call "ScanParameters.vi"("MainConfigurationArray"=w245, "Parameter"="ConnectionDSN") -> ("Value"=w243:string)  [unwired: 9 in]
          n223 = call "SQL_StoreCountersMonitor.vi"("Counters Monitor Array"=w236, "SubAssembly"=w237, "LineName"=w240, "ConnectionDSN"=w243) -> ()  [unwired: 8 in]
        }
      }
    }
    frame #1 {
      n224 = while {
        stop <- "stop" stop-if-true
        # "Get current Hour and Date"
        n225 = Get Date/Time In Seconds() -> (seconds since 1Jan1904=w307:timestamp)
        n226 = Format Date/Time String(time format string (%c)="%x %H:%M:%S", seconds (now)=w307) -> (date/time string=w304:string)  [unwired: 1 in]
        n227 = local write "Hour"(w304) -> ()
        n228 = event shown="[0] Timeout" {
          selector: _ -> [_ _ _ _ _ _ _ _ _ _ _ _ _ _ _ _ _ _ _ _ _ _ _ _ _ _ _ _ _ _]
          dyn-events: _ -> [_ _ _ _ _ _ _ _ _ _ _ _ _ _ _ _ _ _ _ _ _ _ _ _ _ _ _ _ _ _]
          timeout: 50 -> [_ _ _ _ _ _ _ _ _ _ _ _ _ _ _ _ _ _ _ _ _ _ _ _ _ _ _ _ _ _]
          event Timeout {
            n229 = event-data() -> ()  [unwired: 1 in, 3 out]
            n230 = stacked-sequence {
              frame #0 {
                # "Continuously store the Current Counters Montior in a File"
                # "Change the status indicator in the Counters Monitor and Send an Email in case any indicator is Red"
                n231 = local read "Counters Monitor Array"() -> (w330:T16)
                n232 = local read "GeneralParametersArray"() -> (w321:cluster{"Parameter":string, "Value":string}[])
                n233 = local read "GeneralParametersArray"() -> (w312:cluster{"Parameter":string, "Value":string}[])
                n234 = local read "GeneralParametersArray"() -> (w320:cluster{"Parameter":string, "Value":string}[])
                n235 = local read "GeneralParametersArray"() -> (w317:cluster{"Parameter":string, "Value":string}[])
                n236 = local read "GeneralParametersArray"() -> (w325:cluster{"Parameter":string, "Value":string}[])
                n237 = local read "ArrayAlarm"() -> (w327:bool[])
                n238 = call "ScanParameters.vi"("MainConfigurationArray"=w321, "Parameter"="SenderMail") -> ("Value"=w316:string)  [unwired: 9 in]
                n239 = call "ScanParameters.vi"("MainConfigurationArray"=w312, "Parameter"="ConnectionDSN") -> ("Value"=w310:string)  [unwired: 9 in]
                n240 = call "ScanParameters.vi"("MainConfigurationArray"=w320, "Parameter"="Password") -> ("Value"=w315:string)  [unwired: 9 in]
                n241 = call "ScanParameters.vi"("MainConfigurationArray"=w317, "Parameter"="Recipients") -> ("Value"=w314:string)  [unwired: 9 in]
                n242 = call "ScanParameters.vi"("MainConfigurationArray"=w325, "Parameter"="EmailsEnabled") -> ("Value"=w323:string)  [unwired: 9 in]
                n243 = local read "PLC Connection Array"() -> (w309:T11)
                n244 = local read "Line Name"() -> (w328:string)
                n245 = local read "OnlineStations"() -> (w313:T15)
                n246 = call "CountersVisualization.vi"("Counters Monitor Array IN"=w330, "SenderMail"=w316, "ConnectionDSN"=w310, "Password"=w315, "Recipients"=w314, "ArrayAlarmIN"=w327, "LineName"=w328, "PLC Connection Array"=w309, "OnlineStations"=w313, "EmailsEnabled"=w323) -> ("Counters Monitor Array OUT"=w329:T16, "ArrayAlarmOUT"=w326:bool[])  [unwired: 8 in]
                n247 = local write "Counters Monitor Array"(w329) -> ()
                n248 = local write "ArrayAlarm"(w326) -> ()
                n249 = local read "Counters Monitor Array"() -> (w331:T16)
                n250 = local read "CurrentCountersPath"() -> (w333:path)
                n251 = Flatten To JSON(anything=w331) -> (JSON string=w332:string)  [unwired: 2 in, 1 out]
                n252 = call "SaveParameters.vi"("JSON_Text"=w332, "ShiftConfigPath"=w333) -> ()  [unwired: 10 in]
              }
              frame #1 {
                # "If the usser logged in is level 5, enables all the configurations"
                n253 = local read "UserLevel"() -> (w337:i32)
                n254 = Equal?(x=w337, y=5) -> (x = y?=w335:bool)
                n255 = property on="GeneralParametersArray" class="Arr (strict)"("Visible"=w335) -> ()  [unwired: 2 in, 2 out]
                n256 = property on="CreateTables" class="Bool"("Visible"=w335) -> ()  [unwired: 2 in, 2 out]
                n257 = property on="EditUser" class="Bool"("Visible"=w335) -> ()  [unwired: 2 in, 2 out]
                n258 = property on="LoadDefaultConfig" class="Bool"("Visible"=w335) -> ()  [unwired: 2 in, 2 out]
                n259 = property on="ResetAlarmButton" class="Bool"() -> ("Visible"=w334:bool)  [unwired: 2 in, 2 out]
                n260 = case shown="True" w334 {
                  frame False {
                  }
                  frame True {
                    n261 = stacked-sequence {
                      seq-local: [w346 _ _] -> [_ w362 _]
                      seq-local: [w342 _ _] -> [_ w361 _]
                      seq-local: [w339 _ _] -> [_ w360 _]
                      seq-local: [w345 _ _] -> [_ w359 _]
                      frame #0 {
                        n262 = local read "HourResetEnabled"() -> (w350:string)
                        n263 = local read "Hour"() -> (w358:string)
                        n264 = call <vilib>:"Space Constant.vi"() -> ("String"=w357:string)
                        n265 = call <vilib>:"Space Constant.vi"() -> ("String"=w351:string)
                        n266 = Match Pattern(string=w358, regular expression=w357) -> (after substring=w356:string)  [unwired: 1 in, 3 out]
                        n267 = Match Pattern(string=w350, regular expression=w351) -> (after substring=w352:string)  [unwired: 1 in, 3 out]
                        n268 = Match Pattern(string=w356, regular expression=":" ("time format string (%c)")) -> (before substring=w354:string, after substring=w344:string)  [unwired: 1 in, 2 out]
                        n269 = Match Pattern(string=w352, regular expression=":" ("time format string (%c)")) -> (before substring=w340:string, after substring=w338:string)  [unwired: 1 in, 2 out]
                        n270 = Match Pattern(string=w344, regular expression=":" ("time format string (%c)")) -> (before substring=w342:string)  [unwired: 1 in, 3 out]
                        n271 = Decimal String To Number(string=w354) -> (number=w349:i32)  [unwired: 2 in, 1 out]
                        n272 = Decimal String To Number(string=w340) -> (number=w348:i32)  [unwired: 2 in, 1 out]
                        n273 = Match Pattern(string=w338, regular expression=":" ("time format string (%c)")) -> (before substring=w339:string)  [unwired: 1 in, 3 out]
                        n274 = Subtract(x=w349, y=w348) -> (x-y=w345:i32)
                        n275 = Equal?(x=w345, y=0) -> (x = y?=w346:bool)
                      }
                      frame #1 {
                        # "Difference in hours"
                        # "Enabled minute"
                        # "Current minute"
                        n276 = case shown="True" w362 {
                          tunnel: w361 -> [w371 w389]
                          tunnel: w360 -> [w372 w388]
                          tunnel: w359 -> [w378 _]
                          frame False {
                            n277 = Match Pattern(string=w372, regular expression=":" ("time format string (%c)")) -> (before substring=w375:string)  [unwired: 1 in, 3 out]
                            n278 = Match Pattern(string=w371, regular expression=":" ("time format string (%c)")) -> (before substring=w376:string)  [unwired: 1 in, 3 out]
                            n279 = Multiply(x=w378, y=60) -> (x*y=w369:i32)
                            n280 = Decimal String To Number(string=w375) -> (number=w370:i32)  [unwired: 2 in, 1 out]
                            n281 = Decimal String To Number(string=w376) -> (number=w368:i32)  [unwired: 2 in, 1 out]
                            n282 = Subtract(x=w369, y=w370) -> (x-y=w367:i32)
                            n283 = Add(x=w367, y=w368) -> (x+y=w366:i32)
                            n284 = Greater Or Equal?(x=5 ("y"), y=w366) -> (x >= y?=w364:bool)
                            n285 = Not(x=w364) -> (.not. x?=w363:bool)
                            n286 = property on="ResetAlarmButton" class="Bool"("Visible"=w363) -> ()  [unwired: 2 in, 2 out]
                          }
                          frame True {
                            n287 = Match Pattern(string=w389, regular expression=":" ("time format string (%c)")) -> (before substring=w386:string)  [unwired: 1 in, 3 out]
                            n288 = Match Pattern(string=w388, regular expression=":" ("time format string (%c)")) -> (before substring=w385:string)  [unwired: 1 in, 3 out]
                            n289 = Decimal String To Number(string=w386) -> (number=w384:i32)  [unwired: 2 in, 1 out]
                            n290 = Decimal String To Number(string=w385) -> (number=w383:i32)  [unwired: 2 in, 1 out]
                            n291 = Subtract(x=w384, y=w383) -> (x-y=w381:i32)
                            n292 = Greater Or Equal?(x=w381, y=5) -> (x >= y?=w380:bool)
                            n293 = Not(x=w380) -> (.not. x?=w379:bool)
                            n294 = property on="ResetAlarmButton" class="Bool"("Visible"=w379) -> ()  [unwired: 2 in, 2 out]
                          }
                        }
                      }
                      frame #2 {
                        n295 = property on="ResetAlarmButton" class="Bool"() -> ("Visible"=w391:bool)  [unwired: 2 in, 2 out]
                        n296 = case shown="False" w391 {
                          frame False {
                            n297 = local read "GeneralParametersArray"() -> (w399:cluster{"Parameter":string, "Value":string}[])
                            n298 = local read "GeneralParametersArray"() -> (w398:cluster{"Parameter":string, "Value":string}[])
                            n299 = local read "GeneralParametersArray"() -> (w404:cluster{"Parameter":string, "Value":string}[])
                            n300 = call "ScanParameters.vi"("MainConfigurationArray"=w399, "Parameter"="LineName") -> ("Value"=w400:string)  [unwired: 9 in]
                            n301 = call "ScanParameters.vi"("MainConfigurationArray"=w398, "Parameter"="SubAssembly") -> ("Value"=w401:string)  [unwired: 9 in]
                            n302 = Concatenate Strings("update \"", w400, "_userlogged\" set \"useroperations\"='0',\"userquality\"='0' where \"subassembly\"='", w401, "'") -> (w402:string)
                            n303 = call "ScanParameters.vi"("MainConfigurationArray"=w404, "Parameter"="ConnectionDSN") -> ("Value"=w405:string)  [unwired: 9 in]
                            n304 = To Lower Case(string=w402) -> (all lower case string=w403:string)
                            n305 = call "SQL_QueryNoReturn.vi"("SQL query"=w403, "ConnectionDSN"=w405) -> ()  [unwired: 10 in]
                          }
                          frame True {
                          }
                        }
                      }
                    }
                  }
                }
              }
              frame #2 {
                w410 = ":" ("regular expression")
                # "Updates de SQL Table with the current values of the counters monitor each minute"
                n306 = local read "Hour"() -> (w412:string)
                n307 = Match Pattern(string=w412, regular expression=w410) -> (after substring=w411:string)  [unwired: 1 in, 3 out]
                n308 = Match Pattern(string=w411, regular expression=w410) -> (after substring=w409:string)  [unwired: 1 in, 3 out]
                n309 = Decimal String To Number(string=w409) -> (number=w408:i32)  [unwired: 2 in, 1 out]
                n310 = Equal?(x=w408, y=1) -> (x = y?=w407:bool)
                n311 = case shown="True" w407 {
                  frame False {
                  }
                  frame True {
                    n312 = stacked-sequence {
                      frame #0 {
                        n313 = local read "GeneralParametersArray"() -> (w422:cluster{"Parameter":string, "Value":string}[])
                        n314 = local read "GeneralParametersArray"() -> (w416:cluster{"Parameter":string, "Value":string}[])
                        n315 = local read "GeneralParametersArray"() -> (w418:cluster{"Parameter":string, "Value":string}[])
                        n316 = local read "Counters Monitor Array"() -> (w413:T16)
                        n317 = call "ScanParameters.vi"("MainConfigurationArray"=w422, "Parameter"="ConnectionDSN") -> ("Value"=w420:string)  [unwired: 9 in]
                        n318 = call "ScanParameters.vi"("MainConfigurationArray"=w416, "Parameter"="SubAssembly") -> ("Value"=w414:string)  [unwired: 9 in]
                        n319 = call "ScanParameters.vi"("MainConfigurationArray"=w418, "Parameter"="LineName") -> ("Value"=w417:string)  [unwired: 9 in]
                        n320 = call "SQL_CountersMonitorUpdate.vi"("Counters Monitor Array"=w413, "SubAssembly"=w414, "LineName"=w417, "ConnectionDSN"=w420) -> ()  [unwired: 8 in]
                      }
                      frame #1 {
                        n321 = local read "CycleTimeArray"() -> (w425:T1)
                        n322 = local read "LastCycleTimePath"() -> (w423:path)
                        n323 = Flatten To JSON(anything=w425) -> (JSON string=w424:string)  [unwired: 2 in, 1 out]
                        n324 = call "SaveParameters.vi"("JSON_Text"=w424, "ShiftConfigPath"=w423) -> ()  [unwired: 10 in]
                      }
                    }
                  }
                }
              }
            }
          }
          event "SavePLCConfig": Value Change {
            n325 = event-data() -> ()  [unwired: 1 in, 6 out]
            n326 = stacked-sequence {
              frame #0 {
                # "Checks if any parameter was changed and stores the changes in the Modification Array to Store modifications in database"
                n327 = local read "PLC Configuration Path"() -> (w434:path)
                n328 = local read "PLC Connection Array"() -> (w431:T11)
                n329 = local read "UserLogged"() -> (w430:string)
                n330 = call "LoadParameters.vi"("ShiftConfigPath"=w434) -> ("JSON_Text"=w433:string)  [unwired: 10 in]
                n331 = Unflatten From JSON(JSON string=w433, type and defaults=w431) -> (value=w432:T11)  [unwired: 5 in, 1 out]
                n332 = Match Pattern(string=w430, regular expression=",") -> (before substring=w428:string)  [unwired: 1 in, 3 out]
                n333 = for {
                  tunnel: w432 -> [w457] mode=indexing
                  tunnel: w431 -> [w456] mode=indexing
                  tunnel: w428 -> [w439]
                  shift-right: [w435] -> w426
                  shift-left: string[] [] -> [w436]
                  # "Before"
                  n334 = Unbundle By Name(w457) -> ("MachineName"=w454:string, "PLC Address"=w453:string, "PLC Type"=w455:u16, "MemoryNumber1"=w451:string, "MemoryNumber2"=w450:string, "MemoryNumber3"=w449:string)
                  n335 = Unbundle By Name(w456) -> ("MachineName"=w448:string, "PLC Address"=w447:string, "PLC Type"=w446:u16, "MemoryNumber1"=w444:string, "MemoryNumber2"=w443:string, "MemoryNumber3"=w442:string)
                  n336 = Number To Decimal String(number=w455) -> (decimal integer string=w452:string)  [unwired: 1 in]
                  n337 = Number To Decimal String(number=w446) -> (decimal integer string=w445:string)  [unwired: 1 in]
                  n338 = Build Array(w454, w453, w452, w451, w450, w449) -> (w438:string[])
                  n339 = Build Array(w448, w447, w445, w444, w443, w442) -> (w437:string[])
                  n340 = Not Equal?(x=w438, y=w437) -> (x != y?=w441:bool[])
                  n341 = Or Array Elements(Boolean array=w441) -> (logical OR=w440:bool)
                  n342 = case shown="True" w440 {
                    tunnel: w439 -> [_ w460]
                    tunnel: w438 -> [_ w462]
                    tunnel: w437 -> [_ w461]
                    tunnel: [w458 w459] -> w435
                    tunnel: w436 -> [w458 w463]
                    frame False {
                    }
                    frame True {
                      n343 = call "SQL_SortModifications.vi"("UserLogged"=w460, "AfterArray"=w461, "BeforeArray"=w462, "CleanArray"=w463) -> ("ResultArray"=w459:string[])  [unwired: 7 in]
                    }
                  }
                }
                n344 = local write "ModificationArray"(w426) -> ()
              }
              frame #1 {
                n345 = Get Date/Time In Seconds() -> (seconds since 1Jan1904=w468:timestamp)
                n346 = local read "UserLogged"() -> (w471:string)
                n347 = local read "ModificationArray"() -> (w472:string[])
                n348 = Format Date/Time String(time format string (%c)="%x", seconds (now)=w468) -> (date/time string=w466:string)  [unwired: 1 in]
                n349 = Format Date/Time String(time format string (%c)="%H:%M:%S", seconds (now)=w468) -> (date/time string=w465:string)  [unwired: 1 in]
                n350 = Match Pattern(string=w471, regular expression=",") -> (before substring=w464:string)  [unwired: 1 in, 3 out]
                n351 = for {
                  tunnel: w472 -> [w476] mode=indexing
                  tunnel: w466 -> [w480]
                  tunnel: w465 -> [w479]
                  tunnel: w464 -> [w478]
                  w477 = "','"
                  n352 = local read "GeneralParametersArray"() -> (w484:cluster{"Parameter":string, "Value":string}[])
                  n353 = local read "GeneralParametersArray"() -> (w488:cluster{"Parameter":string, "Value":string}[])
                  n354 = call "ScanParameters.vi"("MainConfigurationArray"=w484, "Parameter"="LineName") -> ("Value"=w482:string)  [unwired: 9 in]
                  n355 = call "ScanParameters.vi"("MainConfigurationArray"=w488, "Parameter"="ConnectionDSN") -> ("Value"=w486:string)  [unwired: 9 in]
                  n356 = Concatenate Strings("insert into \"", w482, "_systemlog\" values('", w480, w477, w479, w477, w478, w477, w476, "')") -> (w474:string)
                  n357 = To Lower Case(string=w474) -> (all lower case string=w473:string)
                  n358 = call "SQL_QueryNoReturn.vi"("SQL query"=w473, "ConnectionDSN"=w486) -> ()  [unwired: 10 in]
                }
              }
              frame #2 {
                # "Store the PLC Configuration in JSON File"
                n359 = local read "PLC Connection Array"() -> (w500:T11)
                n360 = local read "PLC Configuration Path"() -> (w499:path)
                n361 = Flatten To JSON(anything=w500) -> (JSON string=w498:string)  [unwired: 2 in, 1 out]
                n362 = local read "GeneralParametersArray"() -> (w494:cluster{"Parameter":string, "Value":string}[])
                n363 = local read "GeneralParametersArray"() -> (w490:cluster{"Parameter":string, "Value":string}[])
                n364 = call "SaveParameters.vi"("JSON_Text"=w498, "ShiftConfigPath"=w499) -> ()  [unwired: 10 in]
                n365 = call "ScanParameters.vi"("MainConfigurationArray"=w494, "Parameter"="ConnectionDSN") -> ("Value"=w492:string)  [unwired: 9 in]
                n366 = call "ScanParameters.vi"("MainConfigurationArray"=w490, "Parameter"="LineName") -> ("Value"=w489:string)  [unwired: 9 in]
                n367 = for {
                  tunnel: w500 -> [w504] mode=indexing
                  tunnel: [w501] -> w495 mode=indexing
                  tunnel: w492 -> [w503]
                  tunnel: w489 -> [w502]
                  n368 = Unbundle By Name(w504) -> ("MachineName"=w501:string)
                  n369 = disable-structure shown="Disabled" {
                    disable-tunnel: w503 -> [w508 _]
                    disable-tunnel: w502 -> [w506 _]
                    disable-tunnel: w501 -> [w505 _]
                    frame Disabled {
                      n370 = call "SQL_CycleTime_RegisterMachine.vi"("MachineName"=w505, "LineName"=w506, "TableName"="CycleTime", "ConnectionDSN"=w508) -> ()  [unwired: 8 in]
                    }
                    frame Enabled {
                    }
                  }
                }
                n371 = local read "CounterLineName Path"() -> (w496:path)
                n372 = local read "Line Name"() -> (w497:string)
                n373 = call "SaveParameters.vi"("JSON_Text"=w497, "ShiftConfigPath"=w496) -> ()  [unwired: 10 in]
                n374 = property on="MachineNameID" class="Ring (strict)"("Strings []"=w495) -> ()  [unwired: 2 in, 2 out]
                n375 = property on="Selector_MachineSpareParts" class="Ring (strict)"("Strings []"=w495) -> ()  [unwired: 2 in, 2 out]
              }
            }
          }
          event "SaveCountersConfig": Value Change {
            n376 = event-data() -> ()  [unwired: 1 in, 6 out]
            n377 = stacked-sequence {
              frame #0 {
                n378 = local read "ThisAppPath"() -> (w510:path)
                n379 = local read "MachineNameID"() -> (w517:u16)
                n380 = property on="MachineNameID" class="Ring (strict)"() -> ("Strings []"=w516:string[])  [unwired: 2 in, 2 out]
                n381 = Path To String(path=w510) -> (string=w509:string)
                n382 = Index Array(array=w516, index=w517) -> (element=w514:string)
                n383 = Concatenate Strings(w509, "\\Config\\CounterSettingConfiguration_" ("regular expression"), w514, ".txt" ("regular expression")) -> (w515:string)
                n384 = String To Path(string=w515) -> (path=w513:path)
                n385 = local write "Counters Configuration Path"(w513) -> ()
              }
              frame #1 {
                # "Checks if any parameter was changed and stores the changes in the Modification Array to Store modifications in database"
                n386 = local read "Counters Configuration Path"() -> (w526:path)
                n387 = local read "CountersConfigArray"() -> (w523:T5)
                n388 = local read "UserLogged"() -> (w522:string)
                n389 = call "LoadParameters.vi"("ShiftConfigPath"=w526) -> ("JSON_Text"=w525:string)  [unwired: 10 in]
                n390 = Unflatten From JSON(JSON string=w525, type and defaults=w523) -> (value=w524:T5)  [unwired: 5 in, 1 out]
                n391 = Match Pattern(string=w522, regular expression=",") -> (before substring=w520:string)  [unwired: 1 in, 3 out]
                n392 = for {
                  tunnel: w524 -> [w547] mode=indexing
                  tunnel: w523 -> [w546] mode=indexing
                  tunnel: w520 -> [w535]
                  shift-right: [w531] -> w518
                  shift-left: string[] [] -> [w532]
                  # "Before"
                  n393 = Unbundle By Name(w547) -> ("ToolCribPartNumber"=w544:string, "ComponentName"=w543:string, "PreparationAlarmCounter"=w545:dbl, "StoppageAlarmCounter"=w530:dbl)
                  n394 = Unbundle By Name(w546) -> ("ToolCribPartNumber"=w541:string, "ComponentName"=w540:string, "PreparationAlarmCounter"=w539:dbl, "StoppageAlarmCounter"=w528:dbl)
                  n395 = Number To Decimal String(number=w539) -> (decimal integer string=w538:string)  [unwired: 1 in]
                  n396 = Number To Decimal String(number=w528) -> (decimal integer string=w527:string)  [unwired: 1 in]
                  n397 = Number To Decimal String(number=w545) -> (decimal integer string=w542:string)  [unwired: 1 in]
                  n398 = Number To Decimal String(number=w530) -> (decimal integer string=w529:string)  [unwired: 1 in]
                  n399 = Build Array(w544, w543, w542, w529) -> (w534:string[])
                  n400 = Build Array(w541, w540, w538, w527) -> (w533:string[])
                  n401 = Not Equal?(x=w534, y=w533) -> (x != y?=w537:bool[])
                  n402 = Or Array Elements(Boolean array=w537) -> (logical OR=w536:bool)
                  n403 = case shown="True" w536 {
                    tunnel: w535 -> [_ w550]
                    tunnel: w534 -> [_ w552]
                    tunnel: w533 -> [_ w551]
                    tunnel: [w548 w549] -> w531
                    tunnel: w532 -> [w548 w553]
                    frame False {
                    }
                    frame True {
                      n404 = call "SQL_SortModifications.vi"("UserLogged"=w550, "AfterArray"=w551, "BeforeArray"=w552, "CleanArray"=w553) -> ("ResultArray"=w549:string[])  [unwired: 7 in]
                    }
                  }
                }
                n405 = local write "ModificationArray"(w518) -> ()
              }
              frame #2 {
                n406 = Get Date/Time In Seconds() -> (seconds since 1Jan1904=w558:timestamp)
                n407 = local read "UserLogged"() -> (w561:string)
                n408 = local read "ModificationArray"() -> (w562:string[])
                n409 = Format Date/Time String(time format string (%c)="%x", seconds (now)=w558) -> (date/time string=w556:string)  [unwired: 1 in]
                n410 = Format Date/Time String(time format string (%c)="%H:%M:%S", seconds (now)=w558) -> (date/time string=w555:string)  [unwired: 1 in]
                n411 = Match Pattern(string=w561, regular expression=",") -> (before substring=w554:string)  [unwired: 1 in, 3 out]
                n412 = for {
                  tunnel: w562 -> [w566] mode=indexing
                  tunnel: w556 -> [w570]
                  tunnel: w555 -> [w569]
                  tunnel: w554 -> [w568]
                  w567 = "','"
                  n413 = local read "GeneralParametersArray"() -> (w574:cluster{"Parameter":string, "Value":string}[])
                  n414 = local read "GeneralParametersArray"() -> (w578:cluster{"Parameter":string, "Value":string}[])
                  n415 = call "ScanParameters.vi"("MainConfigurationArray"=w574, "Parameter"="LineName") -> ("Value"=w572:string)  [unwired: 9 in]
                  n416 = call "ScanParameters.vi"("MainConfigurationArray"=w578, "Parameter"="ConnectionDSN") -> ("Value"=w576:string)  [unwired: 9 in]
                  n417 = Concatenate Strings("insert into \"", w572, "_systemlog\" values('", w570, w567, w569, w567, w568, w567, w566, "')") -> (w564:string)
                  n418 = To Lower Case(string=w564) -> (all lower case string=w563:string)
                  n419 = call "SQL_QueryNoReturn.vi"("SQL query"=w563, "ConnectionDSN"=w576) -> ()  [unwired: 10 in]
                }
              }
              frame #3 {
                n420 = local read "CountersConfigArray"() -> (w580:T5)
                n421 = local read "Counters Configuration Path"() -> (w579:path)
                n422 = Flatten To JSON(anything=w580) -> (JSON string=w581:string)  [unwired: 2 in, 1 out]
                n423 = call "SaveParameters.vi"("JSON_Text"=w581, "ShiftConfigPath"=w579) -> ()  [unwired: 10 in]
              }
            }
          }
          event "SaveCurrentCounter": Value Change {
            n424 = event-data() -> ()  [unwired: 1 in, 6 out]
            n425 = local read "Counters Monitor Array"() -> (w582:T16)
            n426 = local read "CurrentCountersPath"() -> (w584:path)
            n427 = Flatten To JSON(anything=w582) -> (JSON string=w583:string)  [unwired: 2 in, 1 out]
            n428 = call "SaveParameters.vi"("JSON_Text"=w583, "ShiftConfigPath"=w584) -> ()  [unwired: 10 in]
          }
          event "SaveGeneralConfig": Value Change {
            n429 = event-data() -> ()  [unwired: 1 in, 6 out]
            n430 = stacked-sequence {
              frame #0 {
                # "Checks if any parameter was changed and stores the changes in the Modification Array to Store modifications in database"
                n431 = local read "GeneralParametersArray"() -> (w590:cluster{"Parameter":string, "Value":string}[])
                n432 = local read "GeneralConfigPath"() -> (w593:path)
                n433 = local read "UserLogged"() -> (w589:string)
                n434 = call "LoadParameters.vi"("ShiftConfigPath"=w593) -> ("JSON_Text"=w592:string)  [unwired: 10 in]
                n435 = Unflatten From JSON(JSON string=w592, type and defaults=w590) -> (value=w591:cluster{"Parameter":string, "Value":string}[])  [unwired: 5 in, 1 out]
                n436 = Match Pattern(string=w589, regular expression=",") -> (before substring=w587:string)  [unwired: 1 in, 3 out]
                n437 = for {
                  tunnel: w591 -> [w606] mode=indexing
                  tunnel: w590 -> [w605] mode=indexing
                  tunnel: w587 -> [w598]
                  shift-right: [w594] -> w585
                  shift-left: string[] [] -> [w595]
                  # "Before"
                  n438 = Unbundle By Name(w605) -> ("Parameter"=w602:string, "Value"=w601:string)
                  n439 = Unbundle By Name(w606) -> ("Parameter"=w604:string, "Value"=w603:string)
                  n440 = Build Array(w604, w603) -> (w597:string[])
                  n441 = Build Array(w602, w601) -> (w596:string[])
                  n442 = Not Equal?(x=w597, y=w596) -> (x != y?=w600:bool[])
                  n443 = Or Array Elements(Boolean array=w600) -> (logical OR=w599:bool)
                  n444 = case shown="True" w599 {
                    tunnel: w598 -> [_ w609]
                    tunnel: w597 -> [_ w611]
                    tunnel: w596 -> [_ w610]
                    tunnel: [w607 w608] -> w594
                    tunnel: w595 -> [w607 w612]
                    frame False {
                    }
                    frame True {
                      n445 = call "SQL_SortModifications.vi"("UserLogged"=w609, "AfterArray"=w610, "BeforeArray"=w611, "CleanArray"=w612) -> ("ResultArray"=w608:string[])  [unwired: 7 in]
                    }
                  }
                }
                n446 = local write "ModificationArray"(w585) -> ()
              }
              frame #1 {
                n447 = Get Date/Time In Seconds() -> (seconds since 1Jan1904=w617:timestamp)
                n448 = local read "UserLogged"() -> (w620:string)
                n449 = local read "ModificationArray"() -> (w621:string[])
                n450 = Format Date/Time String(time format string (%c)="%x", seconds (now)=w617) -> (date/time string=w615:string)  [unwired: 1 in]
                n451 = Format Date/Time String(time format string (%c)="%H:%M:%S", seconds (now)=w617) -> (date/time string=w614:string)  [unwired: 1 in]
                n452 = Match Pattern(string=w620, regular expression=",") -> (before substring=w613:string)  [unwired: 1 in, 3 out]
                n453 = for {
                  tunnel: w621 -> [w625] mode=indexing
                  tunnel: w615 -> [w629]
                  tunnel: w614 -> [w628]
                  tunnel: w613 -> [w627]
                  w626 = "','"
                  n454 = local read "GeneralParametersArray"() -> (w633:cluster{"Parameter":string, "Value":string}[])
                  n455 = local read "GeneralParametersArray"() -> (w637:cluster{"Parameter":string, "Value":string}[])
                  n456 = call "ScanParameters.vi"("MainConfigurationArray"=w633, "Parameter"="LineName") -> ("Value"=w631:string)  [unwired: 9 in]
                  n457 = call "ScanParameters.vi"("MainConfigurationArray"=w637, "Parameter"="ConnectionDSN") -> ("Value"=w635:string)  [unwired: 9 in]
                  n458 = Concatenate Strings("insert into \"", w631, "_systemlog\" values('", w629, w626, w628, w626, w627, w626, w625, "')") -> (w623:string)
                  n459 = To Lower Case(string=w623) -> (all lower case string=w622:string)
                  n460 = call "SQL_QueryNoReturn.vi"("SQL query"=w622, "ConnectionDSN"=w635) -> ()  [unwired: 10 in]
                }
              }
              frame #2 {
                n461 = local read "GeneralParametersArray"() -> (w638:cluster{"Parameter":string, "Value":string}[])
                n462 = local read "GeneralConfigPath"() -> (w640:path)
                n463 = Flatten To JSON(anything=w638) -> (JSON string=w639:string)  [unwired: 2 in, 1 out]
                n464 = call "SaveParameters.vi"("JSON_Text"=w639, "ShiftConfigPath"=w640) -> ()  [unwired: 10 in]
              }
              frame #3 {
                n465 = local read "GeneralParametersArray"() -> (w641:cluster{"Parameter":string, "Value":string}[])
                n466 = for {
                  tunnel: w641 -> [w642] mode=indexing
                  n467 = Unbundle By Name(w642) -> ()  [unwired: 2 out]
                }
              }
            }
          }
          event "SaveDictionary": Value Change {
            n468 = event-data() -> ()  [unwired: 1 in, 6 out]
            n469 = local read "DictionaryArray"() -> (w645:T14)
            n470 = local read "PathDictionary"() -> (w643:path)
            n471 = Flatten To JSON(anything=w645) -> (JSON string=w644:string)  [unwired: 2 in, 1 out]
            n472 = call "SaveParameters.vi"("JSON_Text"=w644, "ShiftConfigPath"=w643) -> ()  [unwired: 10 in]
          }
          event "RefreshCountersConfig": Value Change {
            n473 = event-data() -> ()  [unwired: 1 in, 6 out]
            n474 = local read "MachineNameID"() -> (w655:u16)
            n475 = local read "ThisAppPath"() -> (w647:path)
            n476 = property on="MachineNameID" class="Ring (strict)"() -> ("Strings []"=w654:string[])  [unwired: 2 in, 2 out]
            n477 = Path To String(path=w647) -> (string=w646:string)
            n478 = Index Array(array=w654, index=w655) -> (element=w652:string)
            n479 = Concatenate Strings(w646, "\\Config\\CounterSettingConfiguration_" ("regular expression"), w652, ".txt" ("regular expression")) -> (w653:string)
            n480 = String To Path(string=w653) -> (path=w648:path)
            n481 = call <vilib>:"Check if File or Folder Exists.vi"("path"=w648) -> ("file or folder exists?"=w649:bool)  [unwired: 8 in, 2 out]
            n482 = case shown="True" w649 {
              tunnel: w648 -> [_ w659]
              frame False {
                n483 = local write "CountersConfigArray"(T5 [] ("CountersConfigArray")) -> ()
              }
              frame True {
                n484 = local read "CountersConfigArray"() -> (w658:T5)
                n485 = call "LoadParameters.vi"("ShiftConfigPath"=w659) -> ("JSON_Text"=w660:string)  [unwired: 10 in]
                n486 = local write "Counters Configuration Path"(w659) -> ()
                n487 = Unflatten From JSON(JSON string=w660, type and defaults=w658) -> (value=w657:T5)  [unwired: 5 in, 1 out]
                n488 = local write "CountersConfigArray"(w657) -> ()
              }
            }
          }
          event "RefreshPLCConfig": Value Change {
            # "Load PLC Connection Information"
            n489 = event-data() -> ()  [unwired: 1 in, 6 out]
            n490 = local read "PLC Configuration Path"() -> (w662:path)
            n491 = local read "PLC Connection Array"() -> (w663:T11)
            n492 = call "LoadParameters.vi"("ShiftConfigPath"=w662) -> ("JSON_Text"=w661:string)  [unwired: 10 in]
            n493 = Unflatten From JSON(JSON string=w661, type and defaults=w663) -> (value=w664:T11)  [unwired: 5 in, 1 out]
            n494 = local write "PLC Connection Array"(w664) -> ()
          }
          event "RefreshGeneralConfig": Value Change {
            n495 = event-data() -> ()  [unwired: 1 in, 6 out]
            n496 = stacked-sequence {
              frame #0 {
                n497 = local read "GeneralConfigPath"() -> (w668:path)
                n498 = local read "GeneralParametersArray"() -> (w666:cluster{"Parameter":string, "Value":string}[])
                n499 = call "LoadParameters.vi"("ShiftConfigPath"=w668) -> ("JSON_Text"=w667:string)  [unwired: 10 in]
                n500 = Unflatten From JSON(JSON string=w667, type and defaults=w666) -> (value=w665:cluster{"Parameter":string, "Value":string}[])  [unwired: 5 in, 1 out]
                n501 = local write "GeneralParametersArray"(w665) -> ()
              }
              frame #1 {
                n502 = local read "GeneralParametersArray"() -> (w670:cluster{"Parameter":string, "Value":string}[])
                n503 = call "ScanParameters.vi"("MainConfigurationArray"=w670, "Parameter"="LineName") -> ("Value"=w671:string)  [unwired: 9 in]
                n504 = local write "Line Name"(w671) -> ()
              }
            }
          }
          event "RefreshCurrentCounter": Value Change {
            n505 = event-data() -> ()  [unwired: 1 in, 6 out]
            n506 = local read "CurrentCountersPath"() -> (w675:path)
            n507 = local read "Counters Monitor Array"() -> (w673:T16)
            n508 = call "LoadParameters.vi"("ShiftConfigPath"=w675) -> ("JSON_Text"=w674:string)  [unwired: 10 in]
            n509 = Unflatten From JSON(JSON string=w674, type and defaults=w673) -> (value=w672:T16)  [unwired: 5 in, 1 out]
            n510 = local write "Counters Monitor Array"(w672) -> ()
          }
          event "ResetAlarm": Value Change {
            n511 = event-data() -> ()  [unwired: 1 in, 6 out]
            n512 = local read "Counters Monitor Array"() -> (w677:T16)
            n513 = local read "ResetAlarm"() -> (w680:bool[])
            n514 = local read "ArrayAlarm"() -> (w679:bool[])
            n515 = for {
              tunnel: w680 -> [w686] mode=indexing
              tunnel: w679 -> [w683] mode=indexing
              tunnel: [w684] -> w678 mode=indexing
              tunnel: w677 -> [w681] mode=indexing
              tunnel: [w682] -> w676 mode=indexing
              n516 = And(x=w686, y=w683) -> (x .and. y?=w685:bool)
              n517 = case shown="True" w685 {
                tunnel: [w688 FALSE] -> w684
                tunnel: w683 -> [w688 _]
                tunnel: w681 -> [w687 _]
                tunnel: [w687 w692] -> w682
                tunnel: w681 -> [_ w690]
                frame False {
                }
                frame True {
                  n518 = local read "OnlineStations"() -> (w689:T15)
                  n519 = Unbundle By Name(w690) -> ("MachineName"=w691:string)
                  n520 = Bundle By Name(cluster=w690, "CurrentCount"=0) -> (w692:T18)
                  n521 = for {
                    tunnel: w691 -> [w700]
                    tunnel: w689 -> [w702] mode=indexing
                    n522 = Unbundle By Name(w702) -> ("MachineName"=w701:string, "Connection"=w699:bool)
                    n523 = Equal?(x=w699, y=TRUE) -> (x = y?=w697:bool)
                    n524 = Equal?(x=w700, y=w701) -> (x = y?=w696:bool)
                    n525 = And(x=w696, y=w697) -> (x .and. y?=w695:bool)
                    n526 = case shown="True" w695 {
                      tunnel: w700 -> [_ w704]
                      frame False {
                      }
                      frame True {
                        (unwired) 0
                        # "Reset the alarm in the PLC"
                        n527 = local read "PLC Connection Array"() -> (w707:T11)
                        n528 = for {
                          tunnel: w707 -> [w716] mode=indexing
                          tunnel: w704 -> [w714]
                          shift-right: [w711] -> w708
                          shift-left: "" -> [w710]
                          tunnel: [w709] -> w703
                          n529 = Unbundle By Name(w716) -> ("MachineName"=w715:string, "PLC Address"=w712:string, "MemoryNumber2"=w709:string)
                          n530 = Equal?(x=w714, y=w715) -> (x = y?=w713:bool)
                          n531 = case shown="False" w713 {
                            tunnel: w712 -> [_ w718]
                            tunnel: [w717 w718] -> w711
                            tunnel: w710 -> [w717 _]
                            frame False {
                            }
                            frame True {
                            }
                          }
                        }
                        n532 = call "CBM_WriteBool_PLC_Keyence.vi"("Set?"=FALSE, "MemoryNumber"=w703, "PLC_IP"=w708) -> ()  [unwired: 8 in, 1 out]
                      }
                    }
                  }
                }
              }
            }
            n533 = local write "Counters Monitor Array"(w676) -> ()
            n534 = local write "ArrayAlarm"(w678) -> ()
          }
          event "RefreshLists": Value Change {
            # "Load PLC Connection Information"
            n535 = event-data() -> ()  [unwired: 1 in, 6 out]
            n536 = local read "PLC Configuration Path"() -> (w721:path)
            n537 = local read "PLC Connection Array"() -> (w722:T11)
            n538 = call "LoadParameters.vi"("ShiftConfigPath"=w721) -> ("JSON_Text"=w720:string)  [unwired: 10 in]
            n539 = Unflatten From JSON(JSON string=w720, type and defaults=w722) -> (value=w719:T11)  [unwired: 5 in, 1 out]
            n540 = local write "PLC Connection Array"(w719) -> ()
            n541 = for {
              tunnel: w719 -> [w724] mode=indexing
              tunnel: [w725] -> w723 mode=indexing
              n542 = Unbundle By Name(w724) -> ("MachineName"=w725:string)
            }
            n543 = property on="Selector_MachineSpareParts" class="Ring (strict)"("Strings []"=w723) -> ()  [unwired: 2 in, 2 out]
          }
          event "ResetAlarmButton": Value Change {
            n544 = event-data() -> ()  [unwired: 1 in, 6 out]
            n545 = local read "GeneralParametersArray"() -> (w729:cluster{"Parameter":string, "Value":string}[])
            n546 = local read "GeneralParametersArray"() -> (w732:cluster{"Parameter":string, "Value":string}[])
            n547 = local read "Counters Monitor Array"() -> (w736:T16)
            n548 = local read "PLC Connection Array"() -> (w726:T11)
            n549 = local read "OnlineStations"() -> (w737:T15)
            n550 = local read "ArrayAlarm"() -> (w733:bool[])
            n551 = call "ScanParameters.vi"("MainConfigurationArray"=w729, "Parameter"="LineName") -> ("Value"=w727:string)  [unwired: 9 in]
            n552 = call "ScanParameters.vi"("MainConfigurationArray"=w732, "Parameter"="ConnectionDSN") -> ("Value"=w730:string)  [unwired: 9 in]
            n553 = call "ResetAlarm.vi"("LineName"=w727, "ConnectionDSN"=w730, "ArrayAlarmIN"=w733, "PLC Connection Array"=w726, "OnlineStations"=w737, "Counters Monitor Array IN"=w736) -> ("ArrayAlarmOUT"=w734:bool[], "Counters Monitor Array OUT"=w735:T16)  [unwired: 4 in]
            n554 = local write "Counters Monitor Array"(w735) -> ()
            n555 = local write "ArrayAlarm"(w734) -> ()
          }
          event "MachineNameID": Value Change {
            n556 = event-data() -> ()  [unwired: 1 in, 6 out]
            n557 = local read "MachineNameID"() -> (w747:u16)
            n558 = local read "ThisAppPath"() -> (w739:path)
            n559 = property on="MachineNameID" class="Ring (strict)"() -> ("Strings []"=w746:string[])  [unwired: 2 in, 2 out]
            n560 = Path To String(path=w739) -> (string=w738:string)
            n561 = Index Array(array=w746, index=w747) -> (element=w744:string)
            n562 = Concatenate Strings(w738, "\\Config\\CounterSettingConfiguration_" ("regular expression"), w744, ".txt" ("regular expression")) -> (w745:string)
            n563 = String To Path(string=w745) -> (path=w740:path)
            n564 = call <vilib>:"Check if File or Folder Exists.vi"("path"=w740) -> ("file or folder exists?"=w741:bool)  [unwired: 8 in, 2 out]
            n565 = case shown="True" w741 {
              tunnel: w740 -> [_ w751]
              frame False {
                n566 = local write "CountersConfigArray"(T5 [] ("CountersConfigArray")) -> ()
              }
              frame True {
                n567 = local read "CountersConfigArray"() -> (w749:T5)
                n568 = call "LoadParameters.vi"("ShiftConfigPath"=w751) -> ("JSON_Text"=w752:string)  [unwired: 10 in]
                n569 = local write "Counters Configuration Path"(w751) -> ()
                n570 = Unflatten From JSON(JSON string=w752, type and defaults=w749) -> (value=w750:T5)  [unwired: 5 in, 1 out]
                n571 = local write "CountersConfigArray"(w750) -> ()
              }
            }
          }
          event "Count Signal": Value Change {
            n572 = event-data() -> ()  [unwired: 1 in, 6 out]
            n573 = local read "OnlineStations"() -> (w753:T15)
            n574 = local read "Count Signal"() -> (w754:bool[])
            n575 = for {
              tunnel: w754 -> [w756] mode=indexing
              tunnel: w753 -> [w757] mode=indexing
              n576 = Unbundle By Name(w757) -> ("MachineName"=w755:string)
              n577 = case shown="True" w756 {
                tunnel: w755 -> [_ w759]
                frame False {
                }
                frame True {
                  n578 = local read "Counters Monitor Array"() -> (w760:T16)
                  n579 = for {
                    tunnel: w760 -> [w763] mode=indexing
                    tunnel: w759 -> [w766]
                    tunnel: [w761] -> w758 mode=indexing
                    n580 = Unbundle By Name(w763) -> ("MachineName"=w767:string, "CurrentCount"=w764:i32)
                    n581 = Equal?(x=w766, y=w767) -> (x = y?=w765:bool)
                    n582 = case shown="False" w765 {
                      tunnel: w764 -> [w768 w770]
                      tunnel: [w768 w769] -> w762
                      frame False {
                      }
                      frame True {
                        n583 = Increment(x=w770) -> (x+1=w769:i32)
                      }
                    }
                    n584 = Bundle By Name(cluster=w763, "CurrentCount"=w762) -> (w761:T18)
                  }
                  n585 = local write "Counters Monitor Array"(w758) -> ()
                }
              }
            }
          }
          event "Sort": Value Change {
            n586 = event-data() -> ()  [unwired: 1 in, 6 out]
            n587 = local read "Counters Monitor Array"() -> (w780:T16)
            n588 = for {
              tunnel: w780 -> [w790] mode=indexing
              tunnel: [w789] -> w778 mode=indexing
              tunnel: [w788] -> w777 mode=indexing
              tunnel: [w786] -> w776 mode=indexing
              tunnel: [w784] -> w775 mode=indexing
              tunnel: [w782] -> w774 mode=indexing
              tunnel: [w781] -> w773 mode=indexing
              n589 = Unbundle By Name(w790) -> ("MachineName"=w789:string, "ComponentName"=w788:string, "StoppageAlarmCounter"=w787:i32, "CurrentCount"=w785:i32, "StatusColorBox"=w783:u32, "ToolCribPartNumber"=w781:string)
              n590 = Number To Decimal String(number=w783) -> (decimal integer string=w782:string)  [unwired: 1 in]
              n591 = Number To Decimal String(number=w787) -> (decimal integer string=w786:string)  [unwired: 1 in]
              n592 = Number To Decimal String(number=w785) -> (decimal integer string=w784:string)  [unwired: 1 in]
            }
            n593 = property on="Table Control" class="Tbl (strict)"("Column Headers[]"=string[] ["MachineName", "ComponentName", "StoppageCounter", "CurrentCount", "StatusColorBox", "ToolCribPartNumber"]) -> ()  [unwired: 2 in, 2 out]
            n594 = Build Array(w778, w777, w776, w775, w774, w773) -> (w772:string[][])
            n595 = Transpose 2D Array(2D array=w772) -> (transposed array=w771:string[][])
            n596 = local write "Table Control"(w771) -> ()
          }
          event "Selector_MachineSpareParts": Value Change {
            n597 = event-data() -> ()  [unwired: 1 in, 6 out]
            n598 = local read "Selector_MachineSpareParts"() -> (w800:u16)
            n599 = property on="Selector_MachineSpareParts" class="Ring (strict)"() -> ("Strings []"=w793:string[])  [unwired: 2 in, 2 out]
            n600 = local read "ThisAppPath"() -> (w792:path)
            n601 = Index Array(array=w793, index=w800) -> (element=w798:string)
            n602 = Path To String(path=w792) -> (string=w791:string)
            n603 = Concatenate Strings(w791, "\\Config\\CounterSettingConfiguration_" ("regular expression"), w798, ".txt" ("regular expression")) -> (w799:string)
            n604 = String To Path(string=w799) -> (path=w796:path)
            n605 = call <vilib>:"Check if File or Folder Exists.vi"("path"=w796) -> ("file or folder exists?"=w797:bool)  [unwired: 8 in, 2 out]
            n606 = case shown="True" w797 {
              tunnel: w796 -> [_ w805]
              frame False {
                n607 = local write "CountersConfigArray"(T5 [] ("CountersConfigArray")) -> ()
              }
              frame True {
                n608 = local read "CountersConfigArray"() -> (w804:T5)
                n609 = call "LoadParameters.vi"("ShiftConfigPath"=w805) -> ("JSON_Text"=w806:string)  [unwired: 10 in]
                n610 = Unflatten From JSON(JSON string=w806, type and defaults=w804) -> (value=w802:T5)  [unwired: 5 in, 1 out]
                n611 = for {
                  tunnel: [w809] -> w803 mode=indexing
                  tunnel: w802 -> [w807] mode=indexing
                  n612 = Unbundle By Name(w807) -> ("ToolCribPartNumber"=w812:string, "ComponentName"=w810:string)
                  n613 = call <vilib>:"Space Constant.vi"() -> ("String"=w808:string)
                  n614 = Concatenate Strings(w812, w808, "-", w808, w810) -> (w809:string)
                }
                n615 = property on="Selector_P#-Description" class="Ring (strict)"("Strings []"=w803) -> ()  [unwired: 2 in, 2 out]
              }
            }
          }
          event "Selector_P#-Description": Value Change {
            n616 = event-data() -> ()  [unwired: 1 in, 6 out]
            n617 = stacked-sequence {
              frame #0 {
                w816 = "_"
                n618 = local read "Selector_MachineSpareParts"() -> (w831:u16)
                n619 = local read "Selector_P#-Description"() -> (w829:u16)
                n620 = property on="Selector_MachineSpareParts" class="Ring (strict)"() -> ("Strings []"=w830:string[])  [unwired: 2 in, 2 out]
                n621 = property on="Selector_P#-Description" class="Ring (strict)"() -> ("Strings []"=w828:string[])  [unwired: 2 in, 2 out]
                n622 = local read "ThisAppPath"() -> (w813:path)
                n623 = Index Array(array=w830, index=w831) -> (element=w824:string)
                n624 = Path To String(path=w813) -> (string=w814:string)
                n625 = Index Array(array=w828, index=w829) -> (element=w821:string)
                n626 = call <vilib>:"Space Constant.vi"() -> ("String"=w820:string)
                n627 = Concatenate Strings(w814, "\\Photos\\Spare Parts\\" ("regular expression")) -> (w822:string)
                n628 = Search and Replace String(input string=w821, search string=w820, replace string="") -> (result string=w818:string)  [unwired: 5 in, 3 out]
                n629 = Search and Replace String(input string=w818, search string="-", replace string=w816) -> (result string=w815:string)  [unwired: 5 in, 3 out]
                n630 = Concatenate Strings(w822, w824, w816, w815, ".jpg") -> (w826:string)
                n631 = String To Path(string=w826) -> (path=w825:path)
                n632 = local write "PathSparePartImage"(w825) -> ()
              }
              frame #1 {
                w835 = "_"
                n633 = local read "Selector_MachineSpareParts"() -> (w850:u16)
                n634 = local read "Selector_P#-Description"() -> (w848:u16)
                n635 = property on="Selector_MachineSpareParts" class="Ring (strict)"() -> ("Strings []"=w849:string[])  [unwired: 2 in, 2 out]
                n636 = property on="Selector_P#-Description" class="Ring (strict)"() -> ("Strings []"=w847:string[])  [unwired: 2 in, 2 out]
                n637 = local read "ThisAppPath"() -> (w833:path)
                n638 = Path To String(path=w833) -> (string=w832:string)
                n639 = Index Array(array=w849, index=w850) -> (element=w843:string)
                n640 = Index Array(array=w847, index=w848) -> (element=w840:string)
                n641 = call <vilib>:"Space Constant.vi"() -> ("String"=w839:string)
                n642 = Concatenate Strings(w832, "\\Photos\\Machine Location\\" ("regular expression")) -> (w841:string)
                n643 = Search and Replace String(input string=w840, search string=w839, replace string="") -> (result string=w837:string)  [unwired: 5 in, 3 out]
                n644 = Search and Replace String(input string=w837, search string="-", replace string=w835) -> (result string=w834:string)  [unwired: 5 in, 3 out]
                n645 = Concatenate Strings(w841, w843, w835, w834, ".jpg") -> (w845:string)
                n646 = String To Path(string=w845) -> (path=w844:path)
                n647 = local write "PathLocationMachineImage"(w844) -> ()
              }
              frame #2 {
                n648 = local read "PathLocationMachineImage"() -> (w851:path)
                n649 = local read "PathSparePartImage"() -> (w854:path)
                n650 = call <vilib>:"Check if File or Folder Exists.vi"("path"=w851) -> ("file or folder exists?"=w852:bool)  [unwired: 8 in, 2 out]
                n651 = call <vilib>:"Check if File or Folder Exists.vi"("path"=w854) -> ("file or folder exists?"=w853:bool)  [unwired: 8 in, 2 out]
                n652 = case shown="True" w852 {
                  tunnel: w851 -> [w855 w863]
                  frame False {
                    n653 = Path To String(path=w855) -> (string=w860:string)
                    n654 = Concatenate Strings("La imagen " ("string"), w860, " no existe." ("string")) -> (w859:string)
                    n655 = One Button Dialog(message=w859, button name ("OK")="OK" ("string")) -> ()  [unwired: 1 out]
                  }
                  frame True {
                    w861 = T20 4 items=["Grayscale (U8)", "Grayscale (I16)", "Grayscale (SGL)", "Complex (CSG)", "RGB (U32)", "HSL (U32)", "RGB (U64)", "Grayscale (U16)"] ("Image Type")
                    n656 = call "IMAQ Create"("Image Name"="LocationInMachine", "Image Type"=w861) -> ("New Image"=w865:T10)  [unwired: 3 in, 1 out]
                    n657 = call "IMAQ ReadFile"("File Path"=w863, "Load Color Palette? (No)"=TRUE, "Image"=w865) -> ("Image Out"=w864:T10)  [unwired: 4 in, 4 out]
                    n658 = local write "Image_LocationInMachine"(w864) -> ()
                  }
                }
                n659 = case shown="True" w853 {
                  tunnel: w854 -> [w871 w878]
                  frame False {
                    n660 = Path To String(path=w871) -> (string=w870:string)
                    n661 = Concatenate Strings("La imagen " ("string"), w870, " no existe." ("string")) -> (w868:string)
                    n662 = One Button Dialog(message=w868, button name ("OK")="OK" ("string")) -> ()  [unwired: 1 out]
                  }
                  frame True {
                    w873 = T20 4 items=["Grayscale (U8)", "Grayscale (I16)", "Grayscale (SGL)", "Complex (CSG)", "RGB (U32)", "HSL (U32)", "RGB (U64)", "Grayscale (U16)"] ("Image Type")
                    n663 = call "IMAQ Create"("Image Name"="SparePart", "Image Type"=w873) -> ("New Image"=w876:T10)  [unwired: 3 in, 1 out]
                    n664 = call "IMAQ ReadFile"("File Path"=w878, "Load Color Palette? (No)"=TRUE, "Image"=w876) -> ("Image Out"=w877:T10)  [unwired: 4 in, 4 out]
                    n665 = local write "Image_SparePart"(w877) -> ()
                  }
                }
              }
            }
          }
          event "GDrive": Value Change {
            n666 = event-data() -> ()  [unwired: 1 in, 6 out]
          }
          event "AddUser": Value Change {
            n667 = event-data() -> ()  [unwired: 1 in, 6 out]
            n668 = local read "GeneralParametersArray"() -> (w884:cluster{"Parameter":string, "Value":string}[])
            n669 = local read "GeneralParametersArray"() -> (w881:cluster{"Parameter":string, "Value":string}[])
            n670 = call "ScanParameters.vi"("MainConfigurationArray"=w884, "Parameter"="ConnectionDSN") -> ("Value"=w880:string)  [unwired: 9 in]
            n671 = call "ScanParameters.vi"("MainConfigurationArray"=w881, "Parameter"="UsersTable") -> ("Value"=w879:string)  [unwired: 9 in]
            n672 = call "SQL_CreateUser.vi"("UsersTable"=w879, "ConnectionDSN"=w880) -> ()  [unwired: 10 in]
          }
          event "RefreshDictionary": Value Change {
            n673 = event-data() -> ()  [unwired: 1 in, 6 out]
            n674 = local read "PathDictionary"() -> (w885:path)
            n675 = call <vilib>:"Check if File or Folder Exists.vi"("path"=w885) -> ("file or folder exists?"=w886:bool)  [unwired: 8 in, 2 out]
            n676 = case shown="True" w886 {
              tunnel: w885 -> [_ w889]
              frame False {
              }
              frame True {
                n677 = local read "DictionaryArray"() -> (w890:T14)
                n678 = call "LoadParameters.vi"("ShiftConfigPath"=w889) -> ("JSON_Text"=w888:string)  [unwired: 10 in]
                n679 = Unflatten From JSON(JSON string=w888, type and defaults=w890) -> (value=w887:T14)  [unwired: 5 in, 1 out]
                n680 = local write "DictionaryArray"(w887) -> ()
              }
            }
          }
          event "Login": Value Change {
            w891 = T19."Enabled" ("Disabled")
            n681 = event-data() -> ()  [unwired: 1 in, 6 out]
            n682 = local read "GeneralParametersArray"() -> (w899:cluster{"Parameter":string, "Value":string}[])
            n683 = local read "GeneralParametersArray"() -> (w898:cluster{"Parameter":string, "Value":string}[])
            n684 = call "ScanParameters.vi"("MainConfigurationArray"=w899, "Parameter"="ConnectionDSN") -> ("Value"=w895:string)  [unwired: 9 in]
            n685 = call "ScanParameters.vi"("MainConfigurationArray"=w898, "Parameter"="UsersTable") -> ("Value"=w894:string)  [unwired: 9 in]
            n686 = property on="PLC Connection Array" class="Arr (strict)"("DisabledEnum"=w891) -> ()  [unwired: 2 in, 2 out]
            n687 = property on="CountersConfigArray" class="Arr (strict)"("DisabledEnum"=w891) -> ()  [unwired: 2 in, 2 out]
            n688 = call "SQL_Login.vi"("UsersTable"=w894, "ConnectionDSN"=w895) -> ("qLevel"=w892:i32, "User"=w893:string)  [unwired: 8 in]
            n689 = local write "UserLevel"(w892) -> ()
            n690 = local write "UserLogged"(w893) -> ()
          }
          event "ShowParetto": Value Change {
            n691 = event-data() -> ()  [unwired: 1 in, 6 out]
          }
          event "LoadDefaultConfig": Value Change {
            n692 = event-data() -> ()  [unwired: 1 in, 6 out]
            n693 = local write "GeneralParametersArray"(cluster{"Parameter":string, "Value":string}[] [{"Parameter"="SenderMail", "Value"="maintenance.nidec.bermudez@gmail.com"}, {"Parameter"="Password", "Value"="Nidec123"}, {"Parameter"="IncidenceRecipients", "Value"="edgar.cruz@nidec.com"}, {"Parameter"="LineName", "Value"="EPSL3"}, {"Parameter"="ConnectionDSN", "Value"="PostgreSQL30"}, {"Parameter"="UsersTable", "Value"="Users"}, {"Parameter"="NidecServer", "Value"="10.110.3.23"}, {"Parameter"="EmailsEnabled", "Value"="Disabled"}] ("GeneralParametersArray")) -> ()
          }
          event "Logout": Value Change {
            w916 = T19."Disabled and Grayed Out" ("Disabled")
            n694 = event-data() -> ()  [unwired: 1 in, 6 out]
            n695 = local write "UserLevel"(0) -> ()
            n696 = local write "UserLogged"("") -> ()
            n697 = property on="PLC Connection Array" class="Arr (strict)"("DisabledEnum"=w916) -> ()  [unwired: 2 in, 2 out]
            n698 = property on="ResetAlarmButton" class="Bool"("Visible"=FALSE) -> ()  [unwired: 2 in, 2 out]
            n699 = property on="CountersConfigArray" class="Arr (strict)"("DisabledEnum"=w916) -> ()  [unwired: 2 in, 2 out]
            n700 = local read "GeneralParametersArray"() -> (w908:cluster{"Parameter":string, "Value":string}[])
            n701 = local read "GeneralParametersArray"() -> (w907:cluster{"Parameter":string, "Value":string}[])
            n702 = local read "GeneralParametersArray"() -> (w913:cluster{"Parameter":string, "Value":string}[])
            n703 = call "ScanParameters.vi"("MainConfigurationArray"=w908, "Parameter"="LineName") -> ("Value"=w909:string)  [unwired: 9 in]
            n704 = call "ScanParameters.vi"("MainConfigurationArray"=w907, "Parameter"="SubAssembly") -> ("Value"=w910:string)  [unwired: 9 in]
            n705 = call "ScanParameters.vi"("MainConfigurationArray"=w913, "Parameter"="ConnectionDSN") -> ("Value"=w914:string)  [unwired: 9 in]
            n706 = Concatenate Strings("update \"", w909, "_userlogged\" set \"useroperations\"='0',\"userquality\"='0' where \"subassembly\"='", w910, "'") -> (w911:string)
            n707 = To Lower Case(string=w911) -> (all lower case string=w912:string)
            n708 = call "SQL_QueryNoReturn.vi"("SQL query"=w912, "ConnectionDSN"=w914) -> ()  [unwired: 10 in]
          }
          event "EditUser": Value Change {
            n709 = event-data() -> ()  [unwired: 1 in, 6 out]
            n710 = local read "GeneralParametersArray"() -> (w924:cluster{"Parameter":string, "Value":string}[])
            n711 = local read "GeneralParametersArray"() -> (w923:cluster{"Parameter":string, "Value":string}[])
            n712 = call "ScanParameters.vi"("MainConfigurationArray"=w924, "Parameter"="ConnectionDSN") -> ("Value"=w919:string)  [unwired: 9 in]
            n713 = call "ScanParameters.vi"("MainConfigurationArray"=w923, "Parameter"="UsersTable") -> ("Value"=w920:string)  [unwired: 9 in]
            n714 = call "SQL_EditUser.vi"("UsersTable"=w920, "ConnectionDSN"=w919) -> ()  [unwired: 8 in, 2 out]
          }
          event "stop": Value Change {
            n715 = event-data() -> ()  [unwired: 1 in, 6 out]
            n716 = Stop() -> ()  [unwired: 1 in]
          }
          event "MaintenanceLogin": Value Change {
            n717 = event-data() -> ()  [unwired: 1 in, 6 out]
            n718 = stacked-sequence {
              seq-local: [w925 _] -> [_ w973]
              frame #0 {
                w929 = ","
                n719 = local read "GeneralParametersArray"() -> (w936:cluster{"Parameter":string, "Value":string}[])
                n720 = local read "GeneralParametersArray"() -> (w935:cluster{"Parameter":string, "Value":string}[])
                n721 = call "ScanParameters.vi"("MainConfigurationArray"=w936, "Parameter"="ConnectionDSN") -> ("Value"=w925:string)  [unwired: 9 in]
                n722 = call "ScanParameters.vi"("MainConfigurationArray"=w935, "Parameter"="UsersTable") -> ("Value"=w934:string)  [unwired: 9 in]
                n723 = call "SQL_Login_Maintenance.vi"("UsersTable"=w934, "ConnectionDSN"=w925) -> ("User"=w931:string)  [unwired: 8 in, 1 out]
                n724 = Match Pattern(string=w931, regular expression=w929) -> (after substring=w930:string)  [unwired: 1 in, 3 out]
                n725 = Match Pattern(string=w930, regular expression=w929) -> (before substring=w928:string)  [unwired: 1 in, 3 out]
                n726 = Equal?(x=w928, y="Maintenance") -> (x = y?=w926:bool)
                n727 = case shown="True" w926 {
                  tunnel: w925 -> [_ w948]
                  frame False {
                  }
                  frame True {
                    n728 = local read "GeneralParametersArray"() -> (w946:cluster{"Parameter":string, "Value":string}[])
                    n729 = local read "GeneralParametersArray"() -> (w945:cluster{"Parameter":string, "Value":string}[])
                    n730 = call "ScanParameters.vi"("MainConfigurationArray"=w946, "Parameter"="SubAssembly") -> ("Value"=w939:string)  [unwired: 9 in]
                    n731 = call "ScanParameters.vi"("MainConfigurationArray"=w945, "Parameter"="LineName") -> ("Value"=w942:string)  [unwired: 9 in]
                    n732 = Concatenate Strings("update \"", w942, "_userlogged\" set \"useroperations\"='1' where \"subassembly\"='", w939, "'") -> (w938:string)
                    n733 = To Lower Case(string=w938) -> (all lower case string=w937:string)
                    n734 = call "SQL_QueryNoReturn.vi"("SQL query"=w937, "ConnectionDSN"=w948) -> ()  [unwired: 10 in]
                  }
                }
              }
              frame #1 {
                w952 = "1"
                n735 = local read "GeneralParametersArray"() -> (w972:cluster{"Parameter":string, "Value":string}[])
                n736 = local read "GeneralParametersArray"() -> (w967:cluster{"Parameter":string, "Value":string}[])
                n737 = call "ScanParameters.vi"("MainConfigurationArray"=w972, "Parameter"="LineName") -> ("Value"=w969:string)  [unwired: 9 in]
                n738 = call "ScanParameters.vi"("MainConfigurationArray"=w967, "Parameter"="SubAssembly") -> ("Value"=w965:string)  [unwired: 9 in]
                n739 = Concatenate Strings("select * from \"" ("SQL query"), w969, "_userlogged\" where \"subassembly\"='", w965, "'") -> (w963:string)
                n740 = To Lower Case(string=w963) -> (all lower case string=w962:string)
                n741 = call "SQL_QueryReturn.vi"("SQL query"=w962, "ConnectionDSN"=w973) -> ("data"=w956:string[][])  [unwired: 9 in]
                n742 = Index Array(array=w956, index (col)=2 ("disabled index (col)")) -> (element=w955:string[])  [unwired: 1 in]
                n743 = Index Array(array=w956, index (col)=1 ("disabled index (col)")) -> (element=w960:string[])  [unwired: 1 in]
                n744 = Index Array(array=w955, index=0 ("disabled index (col)")) -> (element=w953:string)
                n745 = Index Array(array=w960, index=0 ("disabled index (col)")) -> (element=w954:string)
                n746 = Equal?(x=w954, y=w952) -> (x = y?=w951:bool)
                n747 = Equal?(x=w952, y=w953) -> (x = y?=w950:bool)
                n748 = And(x=w951, y=w950) -> (x .and. y?=w949:bool)
                n749 = case shown="True" w949 {
                  tunnel: w949 -> [_ w975]
                  frame False {
                  }
                  frame True {
                    n750 = property on="ResetAlarmButton" class="Bool"("Visible"=w975) -> ()  [unwired: 2 in, 2 out]
                    n751 = local read "Hour"() -> (w974:string)
                    n752 = local write "HourResetEnabled"(w974) -> ()
                  }
                }
              }
            }
          }
          event "QualityLogin": Value Change {
            n753 = event-data() -> ()  [unwired: 1 in, 6 out]
            n754 = stacked-sequence {
              seq-local: [w976 _] -> [_ w1001]
              frame #0 {
                w979 = ","
                n755 = local read "GeneralParametersArray"() -> (w987:cluster{"Parameter":string, "Value":string}[])
                n756 = local read "GeneralParametersArray"() -> (w986:cluster{"Parameter":string, "Value":string}[])
                n757 = call "ScanParameters.vi"("MainConfigurationArray"=w987, "Parameter"="ConnectionDSN") -> ("Value"=w976:string)  [unwired: 9 in]
                n758 = call "ScanParameters.vi"("MainConfigurationArray"=w986, "Parameter"="UsersTable") -> ("Value"=w985:string)  [unwired: 9 in]
                n759 = call "SQL_Login.vi"("UsersTable"=w985, "ConnectionDSN"=w976) -> ("User"=w984:string)  [unwired: 8 in, 1 out]
                n760 = Match Pattern(string=w984, regular expression=w979) -> (after substring=w983:string)  [unwired: 1 in, 3 out]
                n761 = Match Pattern(string=w983, regular expression=w979) -> (before substring=w982:string)  [unwired: 1 in, 3 out]
                n762 = Equal?(x=w982, y="Quality") -> (x = y?=w981:bool)
                n763 = case shown="True" w981 {
                  tunnel: w976 -> [_ w999]
                  frame False {
                  }
                  frame True {
                    n764 = local read "GeneralParametersArray"() -> (w997:cluster{"Parameter":string, "Value":string}[])
                    n765 = local read "GeneralParametersArray"() -> (w996:cluster{"Parameter":string, "Value":string}[])
                    n766 = call "ScanParameters.vi"("MainConfigurationArray"=w997, "Parameter"="SubAssembly") -> ("Value"=w990:string)  [unwired: 9 in]
                    n767 = call "ScanParameters.vi"("MainConfigurationArray"=w996, "Parameter"="LineName") -> ("Value"=w993:string)  [unwired: 9 in]
                    n768 = Concatenate Strings("update \"", w993, "_userlogged\" set \"userquality\"='1' where \"subassembly\"='", w990, "'") -> (w989:string)
                    n769 = To Lower Case(string=w989) -> (all lower case string=w988:string)
                    n770 = call "SQL_QueryNoReturn.vi"("SQL query"=w988, "ConnectionDSN"=w999) -> ()  [unwired: 10 in]
                  }
                }
              }
              frame #1 {
                w1011 = "1"
                n771 = local read "GeneralParametersArray"() -> (w1024:cluster{"Parameter":string, "Value":string}[])
                n772 = local read "GeneralParametersArray"() -> (w1022:cluster{"Parameter":string, "Value":string}[])
                n773 = call "ScanParameters.vi"("MainConfigurationArray"=w1024, "Parameter"="LineName") -> ("Value"=w1023:string)  [unwired: 9 in]
                n774 = call "ScanParameters.vi"("MainConfigurationArray"=w1022, "Parameter"="SubAssembly") -> ("Value"=w1021:string)  [unwired: 9 in]
                n775 = Concatenate Strings("select * from \"" ("SQL query"), w1023, "_userlogged\" where \"subassembly\"='", w1021, "'") -> (w1020:string)
                n776 = To Lower Case(string=w1020) -> (all lower case string=w1019:string)
                n777 = call "SQL_QueryReturn.vi"("SQL query"=w1019, "ConnectionDSN"=w1001) -> ("data"=w1017:string[][])  [unwired: 9 in]
                n778 = Index Array(array=w1017, index (col)=2 ("disabled index (col)")) -> (element=w1016:string[])  [unwired: 1 in]
                n779 = Index Array(array=w1017, index (col)=1 ("disabled index (col)")) -> (element=w1018:string[])  [unwired: 1 in]
                n780 = Index Array(array=w1016, index=0 ("disabled index (col)")) -> (element=w1014:string)
                n781 = Index Array(array=w1018, index=0 ("disabled index (col)")) -> (element=w1015:string)
                n782 = Equal?(x=w1015, y=w1011) -> (x = y?=w1013:bool)
                n783 = Equal?(x=w1011, y=w1014) -> (x = y?=w1012:bool)
                n784 = And(x=w1013, y=w1012) -> (x .and. y?=w1000:bool)
                n785 = case shown="True" w1000 {
                  selector: w1000 -> [_ w1025]
                  frame False {
                  }
                  frame True {
                    n786 = local read "Hour"() -> (w1026:string)
                    n787 = property on="ResetAlarmButton" class="Bool"("Visible"=w1025) -> ()  [unwired: 2 in, 2 out]
                    n788 = local write "HourResetEnabled"(w1026) -> ()
                  }
                }
              }
            }
          }
          event "CreateTables": Value Change {
            n789 = event-data() -> ()  [unwired: 1 in, 6 out]
            n790 = local read "GeneralParametersArray"() -> (w1031:cluster{"Parameter":string, "Value":string}[])
            n791 = local read "GeneralParametersArray"() -> (w1035:cluster{"Parameter":string, "Value":string}[])
            n792 = local read "GeneralParametersArray"() -> (w1029:cluster{"Parameter":string, "Value":string}[])
            n793 = call "ScanParameters.vi"("MainConfigurationArray"=w1031, "Parameter"="LineName") -> ("Value"=w1030:string)  [unwired: 9 in]
            n794 = call "ScanParameters.vi"("MainConfigurationArray"=w1035, "Parameter"="ConnectionDSN") -> ("Value"=w1033:string)  [unwired: 9 in]
            n795 = call "ScanParameters.vi"("MainConfigurationArray"=w1029, "Parameter"="SubAssembly") -> ("Value"=w1027:string)  [unwired: 9 in]
            n796 = call "SQL_CreateTables.vi"("SubAssembly"=w1027, "LineName"=w1030, "ConnectionDSN"=w1033) -> ()  [unwired: 9 in]
          }
        }
      }
      n797 = while {
        stop <- w295 stop-if-true
        # "This loop is in charge of monitor the \nconnection between system and machine"
        n798 = local read "PLC Connection Array"() -> (w293:T11)
        n799 = local read "GeneralParametersArray"() -> (w290:cluster{"Parameter":string, "Value":string}[])
        n800 = for {
          tunnel: w293 -> [w303] mode=indexing
          tunnel: [w300] -> w294 mode=indexing
          tunnel: [w296] -> w292 mode=indexing
          n801 = Unbundle By Name(w303) -> ("MachineName"=w297:string, "PLC Address"=w302:string)
          n802 = local read "CycleTimeCluster"() -> (w299:T6)
          n803 = local read "ConnectionCluster"() -> (w301:cluster{"Connection":bool, "MachineName":string})
          n804 = call "Ping.vi"("hostNameOrAddress"=w302) -> ("bolStatus"=w298:bool)  [unwired: 8 in, 2 out]
          n805 = Bundle By Name(cluster=w301, "MachineName"=w297, "Connection"=w298) -> (w300:cluster{"Connection":bool, "MachineName":string})
          n806 = Bundle By Name(cluster=w299, "MachineName"=w297, "Connection"=w298) -> (w296:T6)
        }
        n807 = call "ScanParameters.vi"("MainConfigurationArray"=w290, "Parameter"="NidecServer") -> ("Value"=w289:string)  [unwired: 9 in]
        n808 = call "Ping.vi"("hostNameOrAddress"=w289) -> ("bolStatus"=w288:bool)  [unwired: 8 in, 2 out]
        n809 = Select(t="Online", s=w288, f="Offline") -> (s? t:f=w287:string)
        n810 = local write "ServerConnectionStatus"(w287) -> ()
        n811 = local write "CycleTimeMonitor"(w292) -> ()
        n812 = local write "OnlineStations"(w294) -> ()
        n813 = local read "stop"() -> (w295:bool)
      }
      n814 = while {
        stop <- w250 stop-if-true
        # "This loop is in charge of couting cycles."
        n815 = local read "Array_BooleanMemoryPLC"() -> (w247:T4)
        n816 = local read "PLC Connection Array"() -> (w248:T11)
        n817 = local read "OnlineStations"() -> (w249:T15)
        n818 = for {
          tunnel: w249 -> [w263] mode=indexing
          tunnel: w248 -> [w261] mode=indexing
          tunnel: w247 -> [w255] mode=indexing
          tunnel: [w252] -> w246 mode=indexing
          # "Count Cycle"
          n819 = Unbundle By Name(w261) -> ("PLC Address"=w259:string, "MemoryNumber1"=w260:string, "MachineName"=w258:string)  [unwired: 1 out]
          n820 = Unbundle By Name(w263) -> ("Connection"=w262:bool)
          n821 = local read "Hour"() -> (w251:string)
          n822 = Unbundle By Name(w255) -> ("PLC_Signal"=w254:bool, "MachineName"=w253:string)
          n823 = case shown="True" w262 {
            tunnel: w260 -> [_ w267]
            tunnel: w259 -> [_ w268]
            tunnel: w258 -> [_ w272]
            tunnel: [w265 w274] -> w257
            tunnel: [w264 w272] -> w256
            tunnel: w254 -> [w265 w275]
            tunnel: w253 -> [w264 w273]
            tunnel: w251 -> [_ w266]
            frame False {
            }
            frame True {
              n824 = call "ReadPLC_Keyence.vi"("MemoryNumber"=w267, "IP Address"=w268) -> ("BoolRead"=w274:bool)  [unwired: 9 in]
              n825 = Equal?(x=w272, y=w273) -> (x = y?=w271:bool)
              n826 = Not Equal?(x=w274, y=w275) -> (x != y?=w270:bool)
              n827 = And(x=w270, y=w271) -> (x .and. y?=w269:bool)
              n828 = case shown="True" w269 {
                tunnel: w274 -> [_ w282]
                tunnel: w272 -> [_ w281]
                tunnel: w266 -> [_ w279]
                frame False {
                }
                frame True {
                  n829 = local read "Counters Monitor Array"() -> (w284:T16)
                  n830 = local read "CycleTimeArray"() -> (w280:T1)
                  n831 = local read "CycleTimeMonitor"() -> (w277:T12)
                  n832 = call "AddCounterWithPLCSignal.vi"("CycleTimeMonitorIN"=w277, "CycleTimeArrayIN"=w280, "Hour"=w279, "Counters Monitor Array IN"=w284, "MachineName"=w281, "PLC_Bool_IN"=w282) -> ("CycleTimeMonitorOUT"=w276:T12, "Counters Monitor Array OUT"=w283:T16, "CycleTimeArrayOUT"=w278:T1)  [unwired: 3 in]
                  n833 = local write "Counters Monitor Array"(w283) -> ()
                  n834 = local write "CycleTimeMonitor"(w276) -> ()
                  n835 = local write "CycleTimeArray"(w278) -> ()
                }
              }
            }
          }
          n836 = Bundle By Name(cluster=w255, "PLC_Signal"=w257, "MachineName"=w256) -> (w252:cluster{"PLC_Signal":bool, "MachineName":string})
        }
        n837 = local write "Array_BooleanMemoryPLC"(w246) -> ()
        n838 = local read "stop"() -> (w250:bool)
      }
    }
  }
